vi "ICDAS_Main.vi"() -> ()   [LabVIEW 2018]
doc: "This is the central application/framework that controls module, run scripts, etc"
uses:
  Framework/InstrumentModulesControl.ctl
  SubVI/VisualizationManagement/PopInOutButton.ctl
  SubVI/Power Request Master 2012 NIVerified/Power Availabilty Requests/Type Defs/Power Request Type.ctl
  NistPluggableModules/BusClass/Bus.lvclass/Bus.ctl
  TypeDefs/PythonOrINIScript.ctl
  LV_Config_class/Typedefs/eLogLvl.ctl
  SubVI/VisualizationManagement/VisualizationManagerActions.ctl
  LV_Config_class/Config.lvclass/Config.ctl
  LV_TestAutomation/Comms_lib/CommsData.ctl
  NistPluggableModules/TestClass/Test.lvclass
  NistPluggableModules/TestClass/Test.lvclass/Test.ctl
  NistPluggableModules/BusClass/Accessors/Read Test.vi
  LV_Config_class/Accessors/Read ConfigFilePath.vi
  NistPluggableModules/TestClass/Accessors/Write ModuleIDs.vi
  <extravilib>/ChannelInstances/Tag-bool/Read With Abort.vi
  <extravilib>/ChannelInstances/Tag-bool/Write With Abort.vi
  <extravilib>/ChannelInstances/Tag-bool/Instantiate.vi
  <extravilib>/ChannelInstances/Tag-bool/EndpointRead.vi
  SubVI/Message Queue/Enqueue Message (Single).vi
  <vilib>/Utility/error.llb/Error Cluster From Error Code.vi
  <extravilib>/ChannelInstances/Tag-bool/Endpoint.vi
  <vilib>/ErrorRing/Error Ring.xnode
  Queue/Queue.lvlib
  <userlib>/NIST/NISTErrorLib/NISTErrorLib.lvlib
  LV_Config_class/Config.lvclass
  <vilib>/Utility/config.llb/NI_LVConfig.lvlib
  LV_Ini/Ini_lib.lvlib
  NistPluggableModules/BusClass/Bus.lvclass
  NistPluggableModules/Visualization/Visualization.lvlib
  LV_TestAutomation/Comms_lib/Comms.lvlib
  <extravilib>/ChannelInstances/Tag-bool.lvlib
  LV_TestAutomation/LV-PY_Lib/LV-PY.lvlib
  NistPluggableModules/Visualization/VisualizeBase/VisualizeBase_class/VisualizeBase.lvclass
  SubVI/Message Queue/Message Queue.lvlib
  SubVI/Power Request Master 2012 NIVerified/Power Requests.lvlib
panel:
  in  "btnRunAll":bool
  in  "btnLoadTDMSData":bool
  in  "btnLoadTDMSData":bool
  in  "btnShutdownICDAS":bool
  in  "btnSettings":bool
  in  "btnHide":bool=TRUE
  in  "rngRunningModules":string(combo)
  in  "btnStopOneModule":bool
  in  "btnPopOutModVis":T1
  in  "ICDAS Logo":enum32{"Page 1"}(tab)
  in  "Visualize":bool
  in  "btnClose Visulizations":bool
  in  "btnPlugins":bool
  in  "Instrument Modules":T2=[{"PluginSelection"=4, "ConfigDialog"=FALSE}] {"PluginSelection" items=["C37.118 PMU", "C37.118 Sim", "Base PMU", "RoomAlert0", "RoomAlert1", "RoomAlert0", "RoomAlert1", "none", "SiemensDEM0"]}
  in  "Experiment Specific Controls":T3(tab)
  in  "Priority":u8=2
  in  "Severity":string="Abort"
  out "COMMS Loop":bool
  in  "RelativePathToINIFiles":string[](array[string])=["..\\UserFiles\\Plugins\\Sensor"]
  in  "Tool Bar?":bool
  out "Error Out":errorcluster
  in  "Severity":string
  in  "Priority":u8=2
  in  "Create Error (Test AutoTimeout)":bool
  in  "Error In 2":errorcluster
  in  "btnCreateScriptlet":bool
  in  "btnRunSpecificScript":bool
  out "CurrentLogFile":string
  # "ICDAS"
  # "Integrated Control and Data Acquisition System"
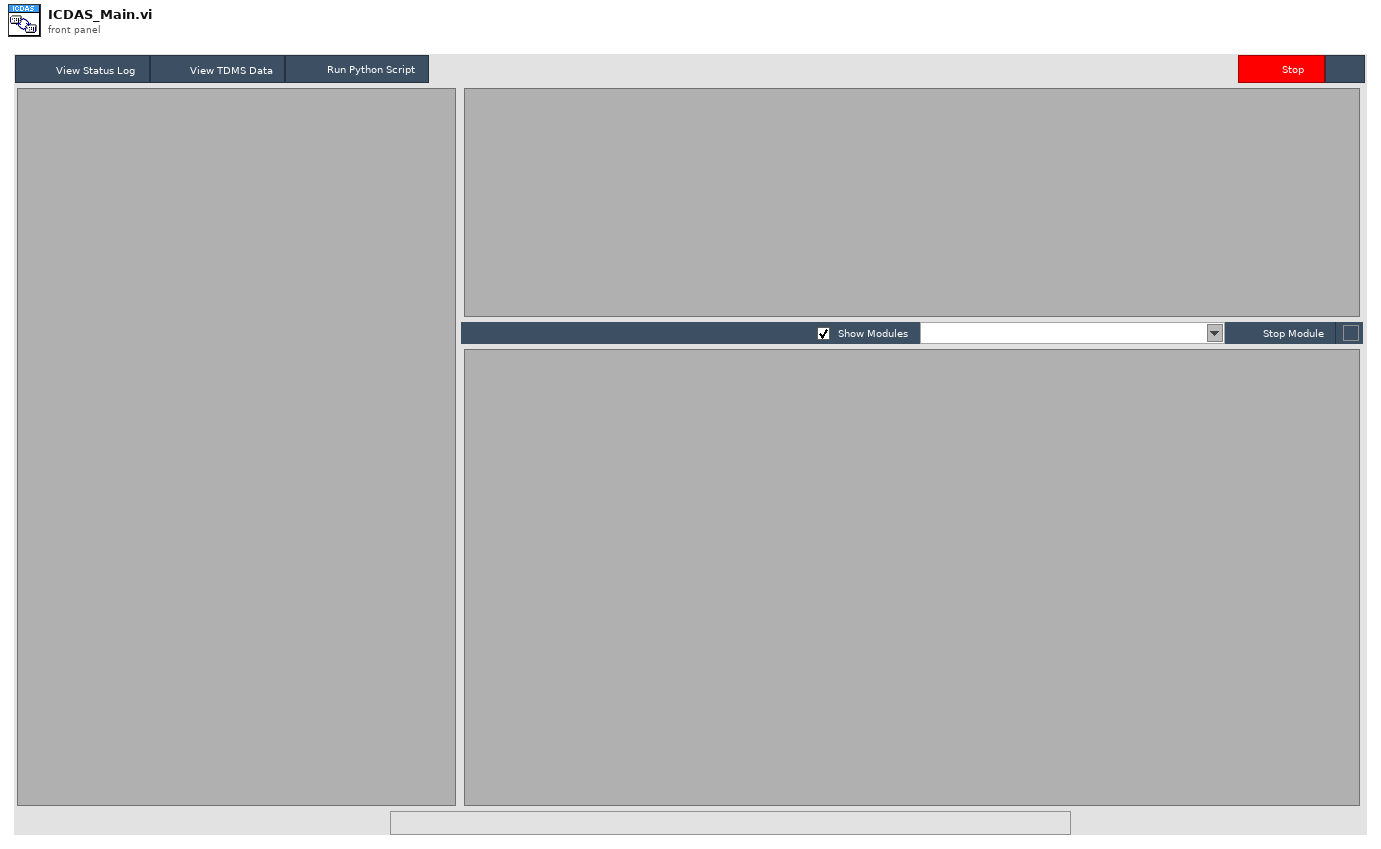
[diagram p1: front panel]
types:
  T1 = typedef "PopInOutButton.ctl" = bool
  T2 = typedef "InstrumentModulesControl.ctl" = cluster{"PluginSelection":u16, "ConfigDialog":bool}[]
  T3 = enum32{"PV Aging Experiment", "Pacific Power ", "Miscellaneous ", "Errors", "Test AutoTimeout", "Test Python MutliRun"}
  T4 = typedef "Power Requests.lvlib/Power Request Type.ctl" = enum32{"Power Request Display Required", "Power Request System Required", "Power Request Away Mode Required", "Power Request Execution Required"}
  T5 = typedef "clUserEvents.ctl" = cluster{"StopEvent":refnum<user-event>, "RefreshUserEvents":refnum<user-event>, "StatusUpdate":refnum<user-event>, "RunAllScripts":refnum<user-event>}
  T6 = typedef "DigitizerShared.lvlib/clBroadcastEvents.ctl" = cluster{"DidInit":refnum<user-event>, "StatusUpdate":refnum<user-event>, "ErrorReport":refnum<user-event>, "DidStop":refnum<user-event>, "PathToINI":refnum<user-event>, "Channels":refnum<user-event>, "Acq":refnum<user-event>, "Trigger":refnum<user-event>, "Waveforms":refnum<user-event>}
  T7 = typedef "FgenShared.lvlib/clBroadcastEvents.ctl" = cluster{"DidInit":refnum<user-event>, "StatusUpdate":refnum<user-event>, "ErrorReport":refnum<user-event>, "DidStop":refnum<user-event>, "PathToINI":refnum<user-event>, "Channels":refnum<user-event>, "Function":refnum<user-event>, "Waveforms":refnum<user-event>, "Triggers":refnum<user-event>, "FunctionParams":refnum<user-event>, "FunctionArbs":refnum<user-event>, "FunctionSampleRate":refnum<user-event>}
  T8 = typedef "SyncModule.lvlib/SyncBroadcastEvents.ctl" = cluster{"DidInit":refnum<user-event>, "StatusUpdate":refnum<user-event>, "ErrorReport":refnum<user-event>, "DidStop":refnum<user-event>, "PathToINI":refnum<user-event>, "TriggerTime":refnum<user-event>, "LockStatus":refnum<user-event>, "Info":refnum<user-event>, "ClockProperties":refnum<user-event>, "SyncData":refnum<user-event>}
  T9 = typedef "AnalysisModule.lvlib/clBroadcastEvents.ctl" = cluster{"DidInit":refnum<user-event>, "StatusUpdate":refnum<user-event>, "ErrorReport":refnum<user-event>, "DidStop":refnum<user-event>, "PathToINI":refnum<user-event>, "Config":refnum<user-event>, "ResultReport":refnum<user-event>, "FunctionClass":refnum<user-event>, "State":refnum<user-event>, "FunctionParams":refnum<user-event>, "Duration":refnum<user-event>}
  T10 = typedef "SensorShared.lvlib/clBroadcastEvents.ctl" = cluster{"DidInit":refnum<user-event>, "StatusUpdate":refnum<user-event>, "ErrorReport":refnum<user-event>, "DidStop":refnum<user-event>, "PathToINI":refnum<user-event>, "SensorReport":refnum<user-event>, "SensorConfig":refnum<user-event>}
  T11 = typedef "ScopeShared.lvlib/clBroadcastEvents.ctl" = cluster{"DidInit":refnum<user-event>, "StatusUpdate":refnum<user-event>, "ErrorReport":refnum<user-event>, "DidStop":refnum<user-event>, "PathToINI":refnum<user-event>, "Handle":refnum<user-event>, "Model":refnum<user-event>, "Channels":refnum<user-event>, "Acquisition":refnum<user-event>, "Trigger":refnum<user-event>, "ExtAcquisition":refnum<user-event>, "Waveform":refnum<user-event>}
  T12 = typedef "AcPwrShared.lvlib/AcPwrBroadcastEvents.ctl" = cluster{"DidInit":refnum<user-event>, "StatusUpdate":refnum<user-event>, "ErrorReport":refnum<user-event>, "DidStop":refnum<user-event>, "PathToINI":refnum<user-event>, "Measurements":refnum<user-event>, "LoadConfigFile":refnum<user-event>, "GetSettings":refnum<user-event>, "SetSettings":refnum<user-event>, "GetType&ID":refnum<user-event>, "GotSettings":refnum<user-event>}
  T13 = cluster{"DigitizerEvents":T6, "FGenEvents":T7, "SyncBroadcastEvents":T8, "AnalysisBroadcastEvents":T9, "SensorBdcstEvents":T10, "ScopeEvents":T11, "clAcPwrEvents":T12}
  T14 = typedef "Visualization.lvlib/VisualizeBase.lvclass/VisBroadcastEvents.ctl" = cluster{"WindowMinimized":refnum<user-event>, "WindowClosed":refnum<user-event>}
  T15 = typedef "cntlRefs.ctl" = cluster{"rngFGen":refnum<vi>, "rngDigitizer":refnum<vi>, "btnHide":refnum<vi>, "rngInst":refnum<vi>, "Instrument Modules":refnum<vi>, "RelativePathToINIFiles ":refnum<vi>, "PluginTree":refnum<vi>, "TestListboxRef":refnum<vi>, "path.tstFile":refnum<vi>, "cmbxRunningModules":refnum<vi>, "TestDataSubPanel":refnum<vi>, "TestDataCaption":refnum<vi>, "btnPopInOut":refnum<vi>, "PluginMgrQ":refnum<queue>, "TestMgrQ":refnum<queue>, "TestMgrSubPanel":refnum<vi>, "PluginMgrSubPanel":refnum<vi>, "PwrReqHandle":u32, "btnStopOneTest":refnum<vi>, "pathUserfiles":refnum<vi>, "PluginTreeCaption":refnum<vi>, "MainVIRef":refnum<vi>}
  T16 = typedef "Comms.lvlib/CommsData.ctl" = cluster{"Command":string, "XMLData":string}
  T17 = typedef "VisualizationManagerActions.ctl" = enum16{"Set", "LoadModVI", "PopInOutModVI", "Add", "Clear", "CloseVisMod", "LoadLatestModule"}
  T18 = typedef "NI_LVConfig.lvlib/Config Data RefNum.ctl" = refnum<k1>
  T19 = typedef "LVBoundsTypeDef.ctl" = cluster{"Width":u32, "Height":u32}
  T20 = typedef "Tag-bool.lvlib/))Channel.ctl" = refnum<queue>
  T21 = typedef "PythonOrINIScript.ctl" = enum16{"INIScript", "Python"}
  T22 = typedef "Config_class.lvlib/Config.lvclass/eLogLvl.ctl" = enum16{"Normal", "Verbose", "None"}
  T23 = enum32{"Invalid", "Standard", "Closed", "Hidden", "Minimized", "Maximized"}
  T24 = typedef "Config_class.lvlib/Config.lvclass/RootDir.ctl" = cluster{"pathRootDir":path, "btnOutPath":bool, "OutDir":string, "btnOpenOutputDir":bool, "ScriptDir":string, "btnOpenScriptDir":bool, "TestDir":string, "btnOpenTestDir":bool}
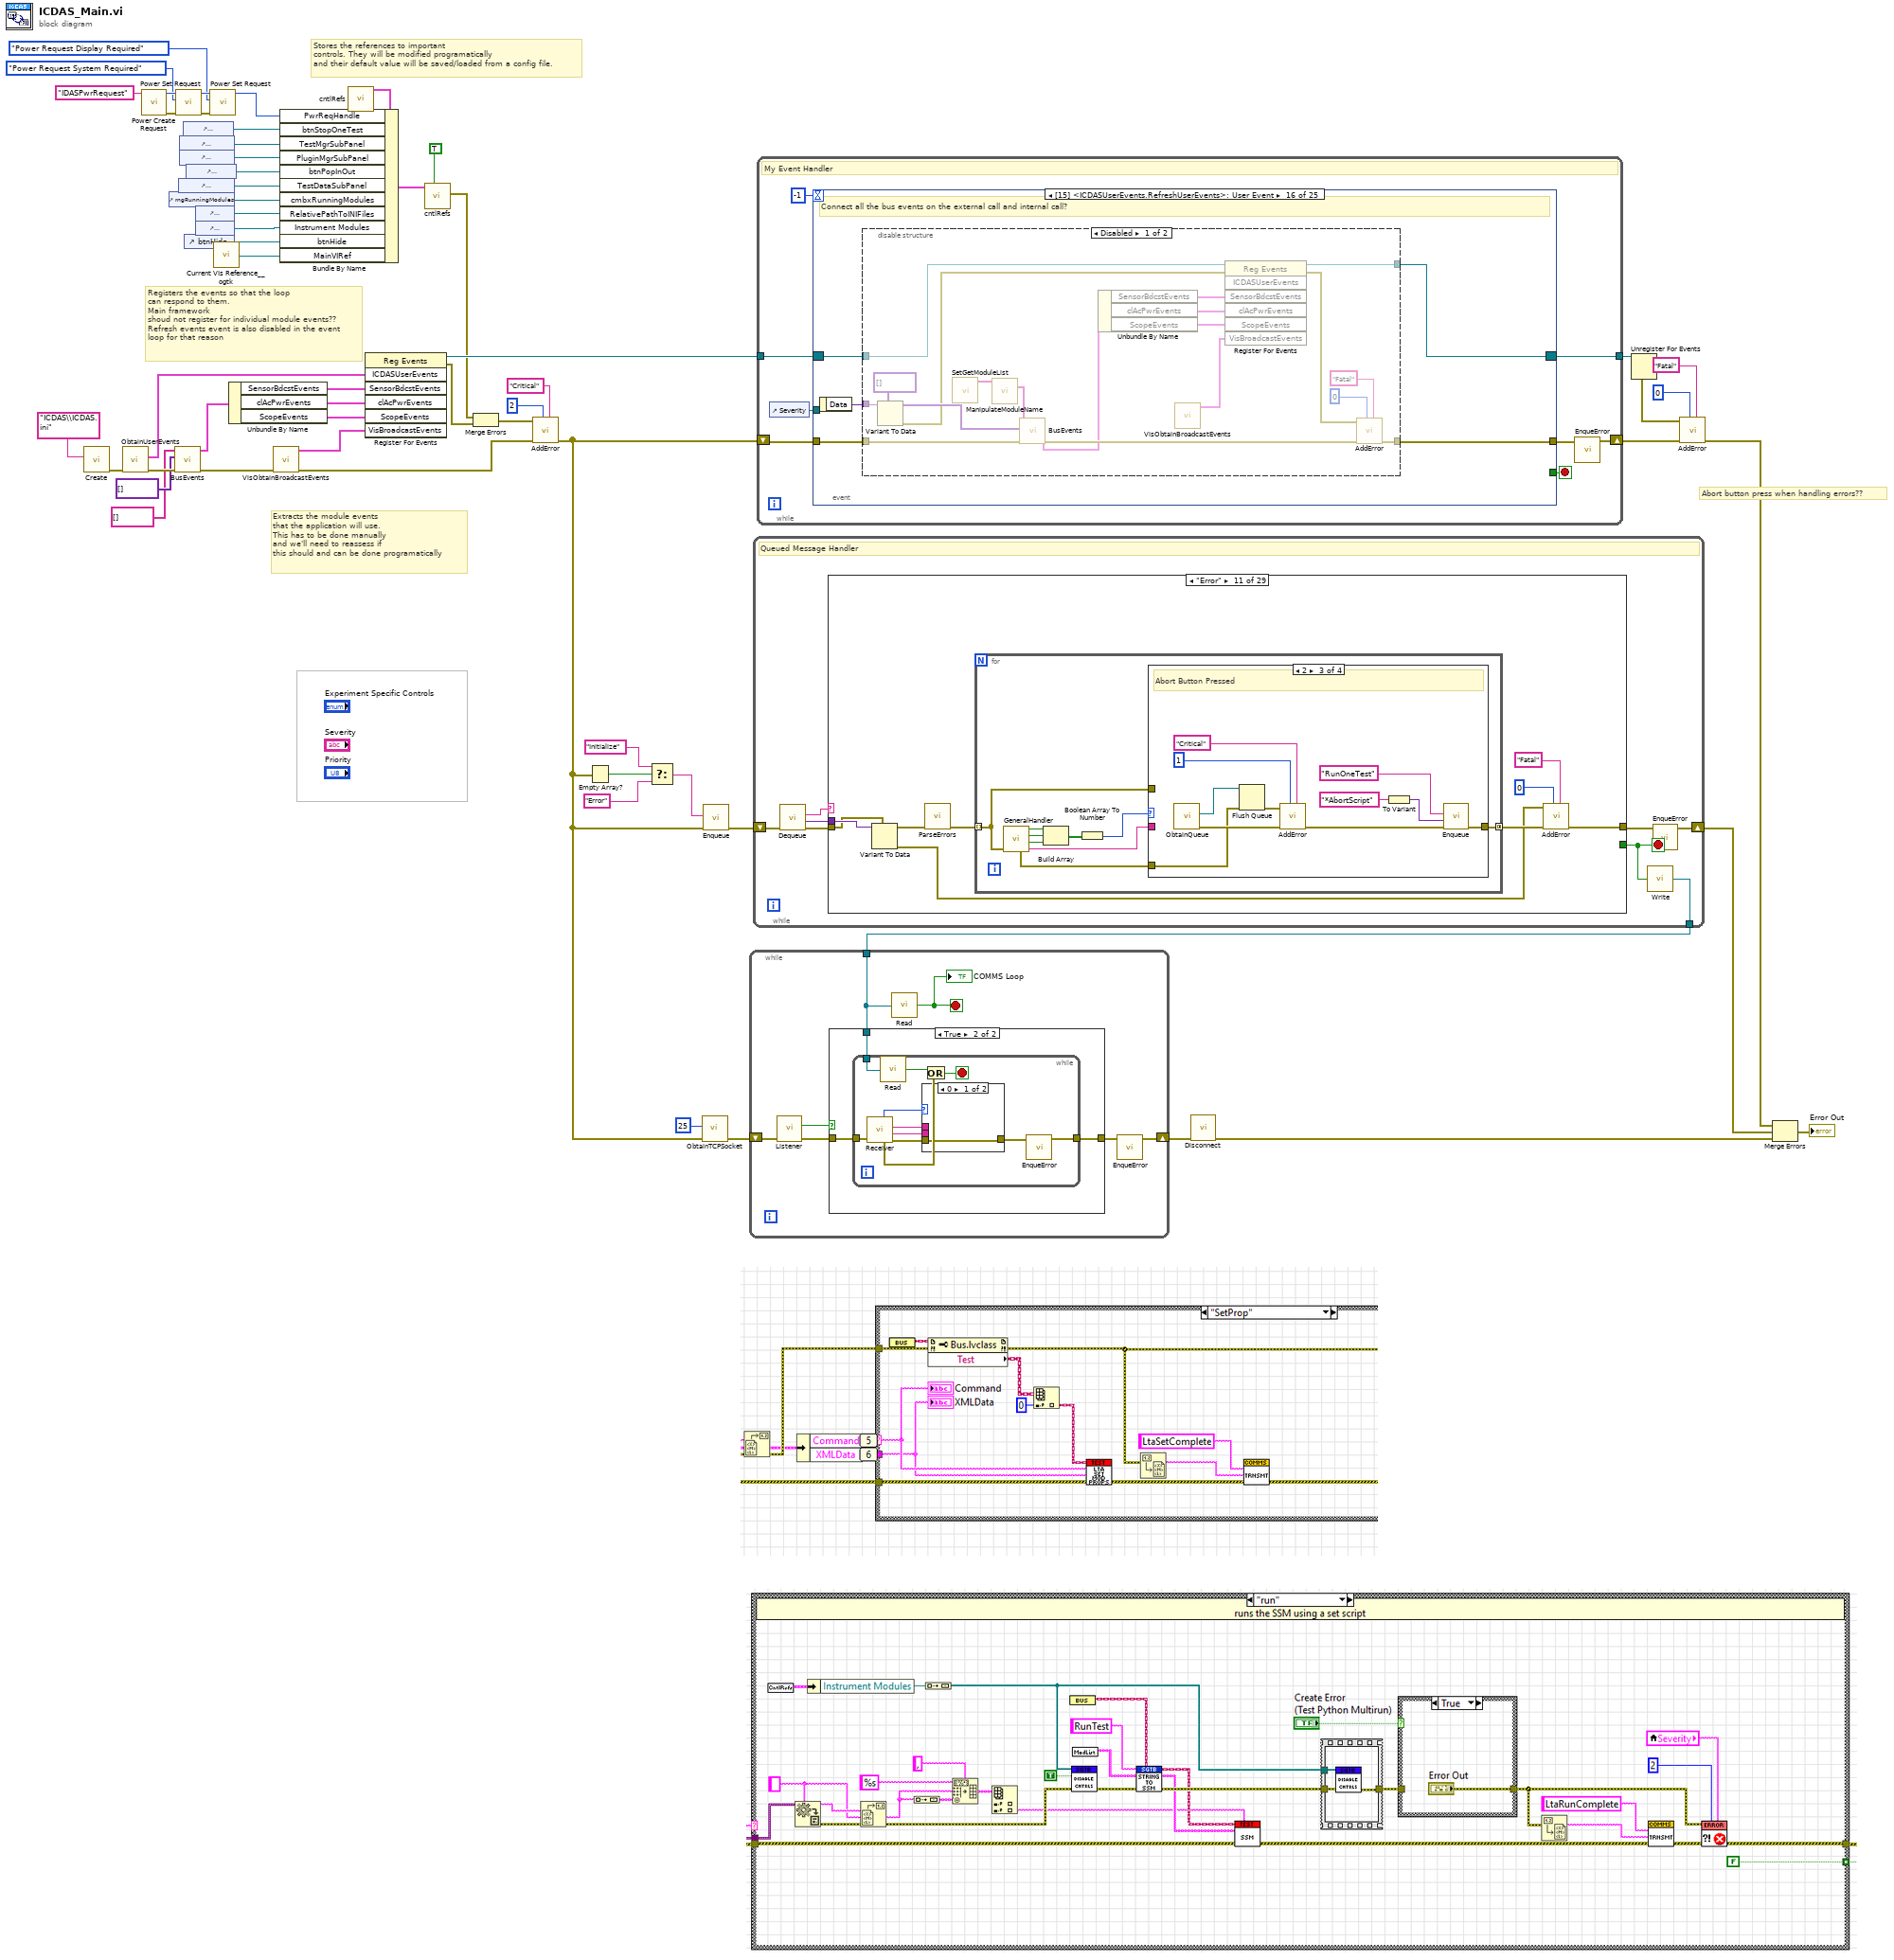
[diagram p0: block diagram]
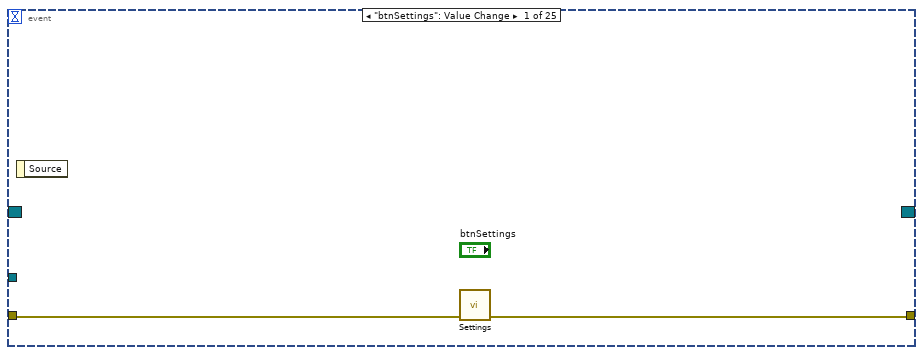
[diagram p2: hidden frame]
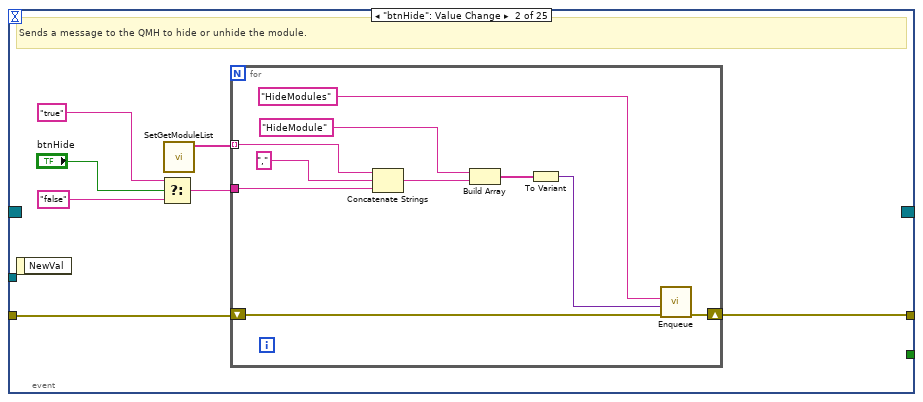
[diagram p3: hidden frame]
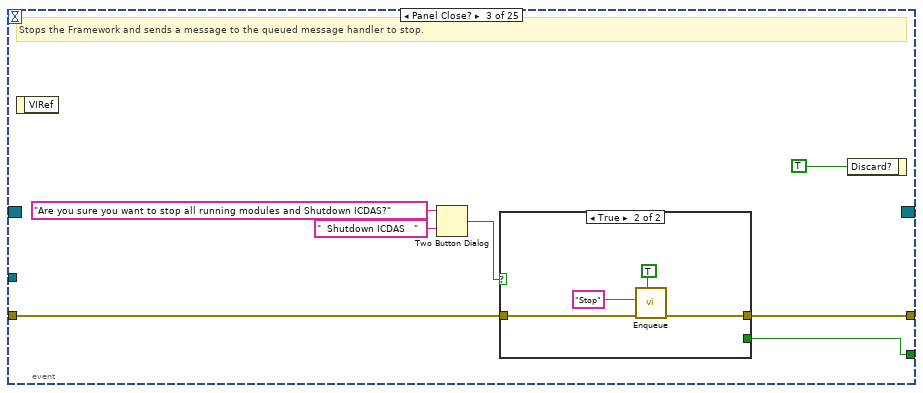
[diagram p4: hidden frame]
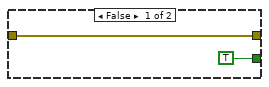
[diagram p5: hidden frame]
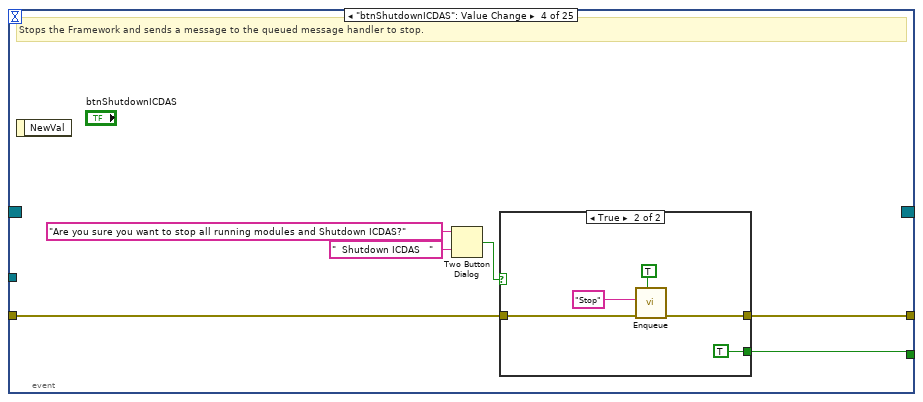
[diagram p6: hidden frame]
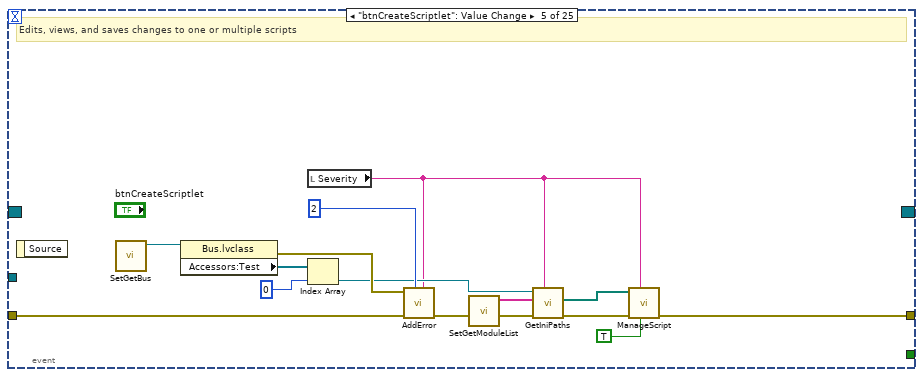
[diagram p8: hidden frame]
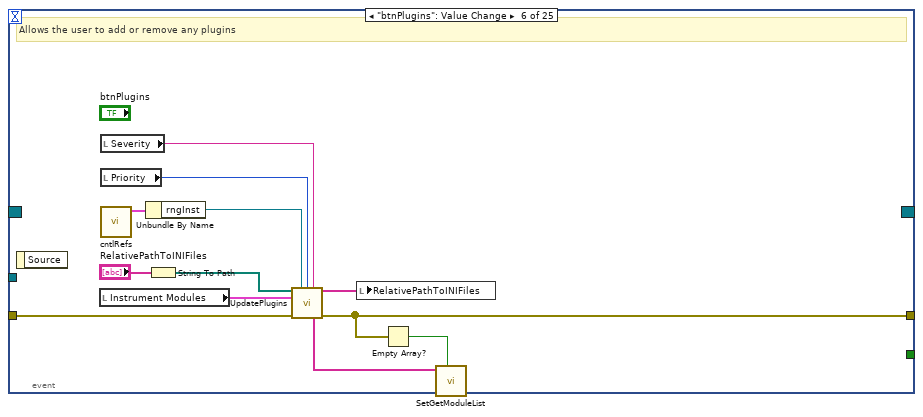
[diagram p9: hidden frame]
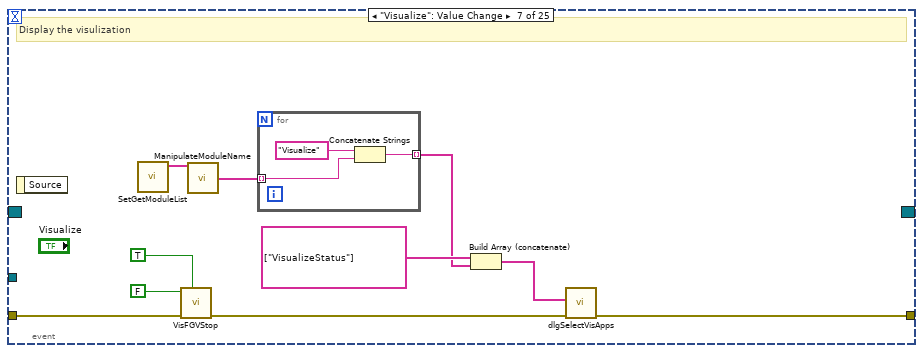
[diagram p10: hidden frame]
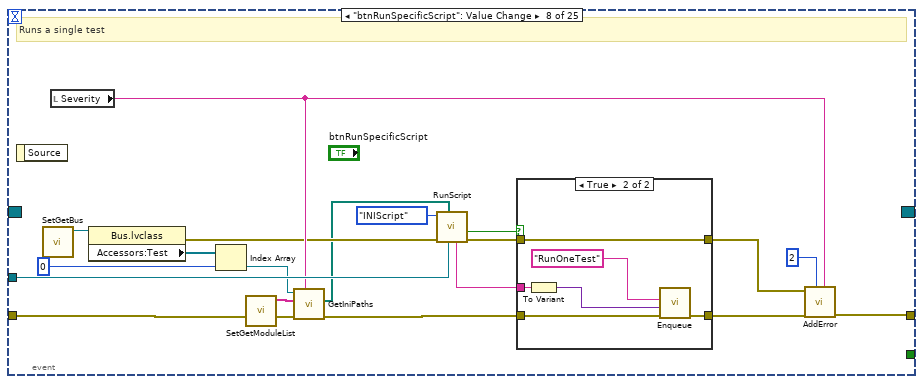
[diagram p11: hidden frame]
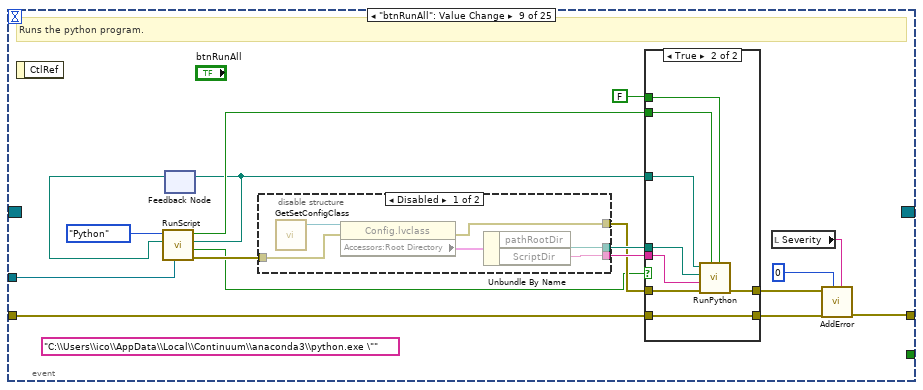
[diagram p13: hidden frame]
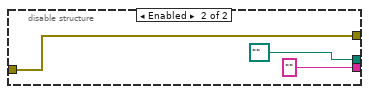
[diagram p15: hidden frame]
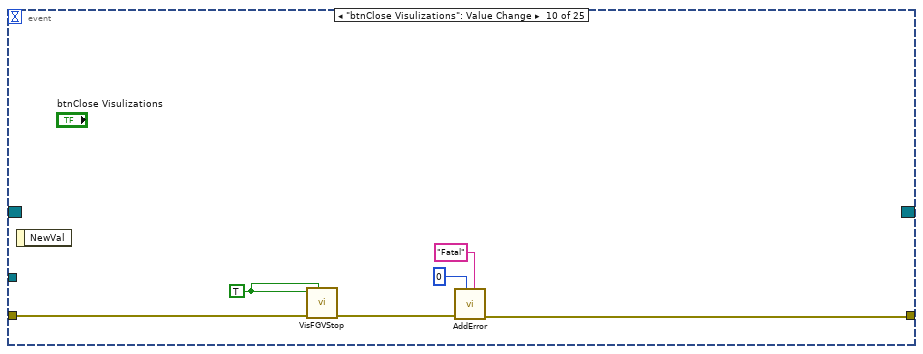
[diagram p16: hidden frame]
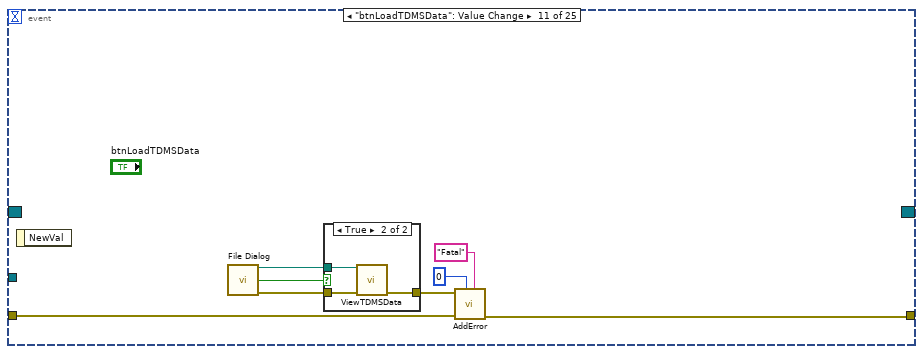
[diagram p17: hidden frame]
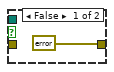
[diagram p18: hidden frame]
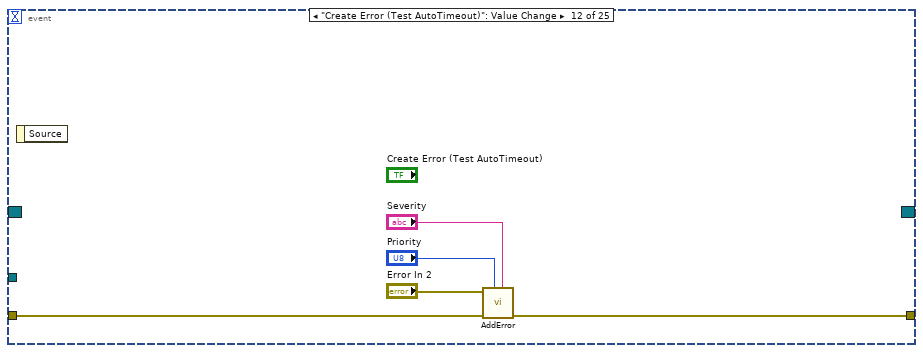
[diagram p19: hidden frame]
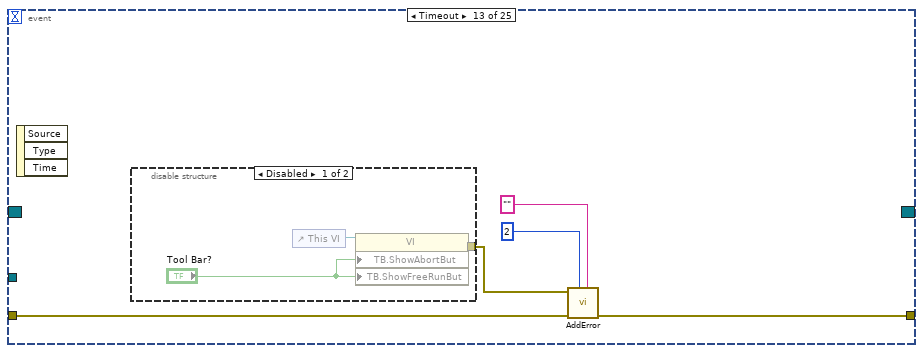
[diagram p20: hidden frame]
diagram:
  # "Abort button press when handling errors??"
  # "Registers the events so that the loop \ncan respond to them.\nMain framework\nshoud not register for individual module events??\nRefresh events event is also disabled in the event \nloop for that reason"
  # "Extracts the module events\nthat the application will use. \nThis has to be done manually \nand we'll need to reassess if \nthis should and can be done programatically"
  # "Stores the references to important\ncontrols. They will be modified programatically\nand their default value will be saved/loaded from a config file."
  n1 = call "Create.vi"("name or relative path"="ICDAS\\ICDAS.ini") -> ("ErrorArray"=w51:errorcluster[])  [unwired: 9 in, 1 out]
  n2 = call "ObtainUserEvents.vi"("ErrorArray"=w51) -> ("ErrorArray"=w52:errorcluster[], "ICDASUserEvents"=w58:T5)  [unwired: 9 in]
  n3 = call "Power Create Request.vi"("Simple Reason String"="IDASPwrRequest") -> ("error out"=w16:errorcluster, "Handle"=w17:i64)  [unwired: 9 in]
  n4 = control-ref of="rngRunningModules"() -> (w25:refnum<vi>)
  n5 = call "BusEvents.vi"("Error in"=w52, "EventArray"=variant[] [], "ModuleList"=string[] []) -> ("Error out"=w9:errorcluster[], "output cluster"=w39:T13)  [unwired: 7 in]
  n6 = call "Power Set Request.vi"("error in (no error)"=w16, "Power Request Type"=Power_Request_Type."Power Request System Required", "Handle in"=w17) -> ("error out"=w14:errorcluster, "Handle out"=w15:u32)  [unwired: 6 in, 1 out]
  n7 = control-ref of="TestDataSubPanel"() -> (w24:refnum<vi>)
  n8 = control-ref of="TestMgrSubPanel"() -> (w19:refnum<vi>)
  n9 = control-ref of="PluginMgrSubPanel"() -> (w20:refnum<vi>)
  n10 = control-ref of="btnStopOneModule"() -> (w10:refnum<vi>)
  n11 = control-ref of="btnHide"() -> (w48:refnum<vi>)
  n12 = control-ref of="btnPopOutModVis"() -> (w23:refnum<vi>)
  n13 = control-ref of="RelativePathToINIFiles"() -> (w34:refnum<vi>)
  n14 = control-ref of="Instrument Modules"() -> (w37:refnum<vi>)
  n15 = call "Power Set Request.vi"("error in (no error)"=w14, "Power Request Type"=Power_Request_Type."Power Request Display Required", "Handle in"=w15) -> ("Handle out"=w11:u32)  [unwired: 6 in, 2 out]
  n16 = call <userlib>:"Current VIs Reference__ogtk.vi"() -> ("Current VI's reference"=w1:refnum<vi>)  [unwired: 5 in]
  n17 = Unbundle By Name(w39) -> ("SensorBdcstEvents"=w38:T10, "clAcPwrEvents"=w4:T12, "ScopeEvents"=w29:T11)
  n18 = call "VisObtainBroadcastEvents.vi"("Error"=w9) -> ("Error"=w8:errorcluster[], "VisBroadcastEvents"=w3:T14)  [unwired: 9 in]
  n19 = call "cntlRefs.vi"() -> ("cntlRefs"=w22:T15)  [unwired: 10 in, 1 out]
  n20 = Bundle By Name(cluster=w22, "PwrReqHandle"=w11, "btnStopOneTest"=w10, "TestMgrSubPanel"=w19, "PluginMgrSubPanel"=w20, "btnPopInOut"=w23, "TestDataSubPanel"=w24, "cmbxRunningModules"=w25, "RelativePathToINIFiles"=w34, "Instrument Modules"=w37, "btnHide"=w48, "MainVIRef"=w1) -> (w41:T15)
  n21 = register-events(w58, w38, w4, w29, w3) -> (reference out=w59:refnum<event-registration>, error out=w28:errorcluster)  [unwired: 2 in]
  n22 = call "cntlRefs.vi"("Set?"=TRUE, "cntlRefs"=w41) -> ("error out"=w26:errorcluster[])  [unwired: 8 in, 1 out]
  n23 = Merge Errors(w26, w28) -> (w27:errorcluster)
  n24 = call <userlib>:"AddError.vi"("Severity"="Critical", "Priority"=u8 2, "ErrorArray In"=w8, "error in (no error)"=w27) -> ("ErrorArray Out"=w40:errorcluster[])  [unwired: 6 in, 1 out]
  n25 = Empty Array?(array=w40) -> (empty?=w56:bool)
  n26 = Select(t="Initialize" ("Message"), s=w56, f="Error") -> (s? t:f=w53:string)
  n27 = call "ObtainTCPSocket.vi"("ErrorArray"=w40, "timeout"=25) -> ("ErrorArray"=w46:errorcluster[])  [unwired: 8 in, 1 out]
  n28 = call "Enqueue.vi"("ErrorArray"=w40, "Message"=w53) -> ("ErrorArray"=w57:errorcluster[])  [unwired: 9 in]
  n29 = while {
    shift-right: [w64] -> w35
    shift-left: w57 -> [w67]
    tunnel: [w60] -> w43
    stop <- w62 stop-if-true
    # "Queued Message Handler"
    n30 = call "Dequeue.vi"("ErrorArray"=w67) -> ("ErrorArray"=w63:errorcluster[], "Message Data"=w61:variant, "Message"=w66:string)  [unwired: 8 in]
    n31 = case shown="\"Error\"" w66 {
      selector: w66 -> [_ _ _ _ _ _ _ _ _ _ _ _ _ _ _ _ w306 _ _ _ _ _ _ _ _ _ _ _ _]
      tunnel: [w68 w82 w91 w107 w129 w130 w137 w153 w214 w216 w218 w249 w256 w262 w283 w297 w305 w314 w329 w331 w338 w341 w347 w352 w354 w361 w371 w375 w397] -> w65
      tunnel: w63 -> [w68 w70 w101 w114 w128 w130 w139 w154 w215 w216 w223 w255 w256 w261 w278 w300 w304 w314 w330 w331 w337 w346 w347 w351 w354 w361 w371 w374 w397]
      tunnel: [_ _ _ _ _ _ _ _ _ _ _ _ _ _ _ TRUE _ _ _ _ _ _ _ _ _ _ _ _ _] -> w62
      tunnel: w61 -> [_ _ _ _ w127 _ w140 w155 _ _ w224 w254 _ _ w282 _ _ _ w327 _ w336 _ _ _ _ _ w365 w381 _]
      frame "----Initialization----" {
      }
      frame "Initialize" {
        # "Pulls the default configuration from the INI file"
        n32 = call "GetSetConfigClass.vi"() -> ("Ref out"=w87:refnum<class "Config.lvclass">)  [unwired: 11 in]
        n33 = property class="Config.lvclass"(reference=w87) -> ("Accessors:ConfigFilePath"=w84:path)  [unwired: 1 in, 2 out]
        n34 = call "Enqueue.vi"("ErrorArray"=w70, "Message"="Load Manager VIs") -> ("ErrorArray"=w69:errorcluster[])  [unwired: 9 in]
        n35 = To Variant(anything=w84) -> (Variant=w83:variant)
        n36 = call "Enqueue.vi"("ErrorArray"=w69, "Message Data"=w83, "Message"="LoadTest") -> ("ErrorArray"=w72:errorcluster[])  [unwired: 8 in]
        n37 = call "ClearBus.vi"("ErrorIn"=w72) -> ("ErrorOut"=w73:errorcluster[])  [unwired: 10 in]
        n38 = call "Enqueue.vi"("ErrorArray"=w73, "Message Data"=FALSE, "Message"="Clear Test Controls") -> ("ErrorArray"=w74:errorcluster[])  [unwired: 8 in]
        n39 = call "Enqueue.vi"("ErrorArray"=w74, "Message Data"=FALSE ("Delete Children?"), "Message"="Show Test Data Controls") -> ("ErrorArray"=w79:errorcluster[])  [unwired: 8 in]
        n40 = call "Enqueue.vi"("ErrorArray"=w79, "Message"="Center Logo") -> ("ErrorArray"=w81:errorcluster[])  [unwired: 9 in]
        n41 = call <userlib>:"AddError.vi"("Severity"="Fatal", "Priority"=u8 0, "ErrorArray In"=w81) -> ("ErrorArray Out"=w82:errorcluster[])  [unwired: 7 in, 1 out]
      }
      frame "Load Manager VIs" {
        # "Load Plugin Manager first..."
        n42 = call "cntlRefs.vi"() -> ("cntlRefs"=w100:T15)  [unwired: 10 in, 1 out]
        n43 = Unbundle By Name(w100) -> ("PluginMgrSubPanel"=w95:refnum<vi>)
        n44 = vi-ref "PluginManager.vi"() -> (w96:refnum<vi>)
        n45 = invoke class="VI" method="FP.Close"(reference=w96) -> (reference out=w97:refnum<vi>)  [unwired: 2 in, 2 out]
        n46 = invoke class="VI" method="Run VI"(reference=w97, "Wait until done"=FALSE ("Wait Until Done"), "Auto Dispose Ref"=FALSE ("Auto Dispose Reference")) -> (reference out=w93:refnum<vi>, error out=w94:errorcluster)  [unwired: 2 in, 3 out]
        n47 = invoke class="SubPnl" method="Insert VI"(reference=w95, error in=w94, "VI Ref"=w93) -> (error out=w92:errorcluster)  [unwired: 1 in, 3 out]
        n48 = call <userlib>:"AddError.vi"("Severity"="Fatal", "Priority"=u8 0, "ErrorArray In"=w101, "error in (no error)"=w92) -> ("ErrorArray Out"=w91:errorcluster[])  [unwired: 6 in, 1 out]
      }
      frame "Plugin Manager Loaded" {
        # "Load Test Manager after plugin manager has been loaded"
        n49 = vi-ref "TestManager.vi"() -> (w113:refnum<vi>)
        n50 = call "cntlRefs.vi"() -> ("cntlRefs"=w104:T15)  [unwired: 10 in, 1 out]
        n51 = invoke class="VI" method="FP.Close"(reference=w113) -> (reference out=w112:refnum<vi>)  [unwired: 2 in, 2 out]
        n52 = Unbundle By Name(w104) -> ("TestMgrSubPanel"=w103:refnum<vi>)
        n53 = invoke class="VI" method="Run VI"(reference=w112, "Wait until done"=FALSE ("Wait Until Done"), "Auto Dispose Ref"=FALSE ("Auto Dispose Reference")) -> (reference out=w111:refnum<vi>, error out=w110:errorcluster)  [unwired: 2 in, 3 out]
        n54 = invoke class="SubPnl" method="Insert VI"(reference=w103, error in=w110, "VI Ref"=w111) -> (error out=w102:errorcluster)  [unwired: 1 in, 3 out]
        n55 = call <userlib>:"AddError.vi"("Severity"="Critical", "Priority"=u8 2, "ErrorArray In"=w114, "error in (no error)"=w102) -> ("ErrorArray Out"=w107:errorcluster[])  [unwired: 6 in, 1 out]
      }
      frame "LoadTest" {
        # "From the default file load the last saved results and updated the controls and indicators"
        n56 = call "cntlRefs.vi"() -> ("cntlRefs"=w121:T15)  [unwired: 10 in, 1 out]
        n57 = Unbundle By Name(w121) -> ("btnHide"=w120:refnum<vi>)
        n58 = Variant To Data(type=path "", Variant=w127) -> (data=w123:path, error out=w125:errorcluster)  [unwired: 1 in]
        n59 = call <vilib>:"Open Config Data.vi"("error in (no error)"=w125, "configuration file path"=w123) -> ("error out"=w117:errorcluster, "refnum"=w122:T18)  [unwired: 7 in, 1 out]
        n60 = Build Array(w120) -> (w119:refnum<vi>[])
        n61 = call "InitBoolValues.vi"("ErrorArray in"=w128, "BoolRefArray"=w119, "IniFileRef in"=w122) -> ("ErrorArray Out"=w126:errorcluster[], "IniFileRef out"=w118:T18)  [unwired: 7 in]
        n62 = call <vilib>:"Close Config Data.vi"("error in (no error)"=w117, "refnum"=w118) -> ("error out"=w116:errorcluster)  [unwired: 8 in, 1 out]
        n63 = call <userlib>:"AddError.vi"("Severity"="Inform", "ErrorArray In"=w126, "error in (no error)"=w116) -> ("ErrorArray Out"=w129:errorcluster[])  [unwired: 7 in, 1 out]
      }
      frame "----Python Communications----" {
      }
      frame "get" {
        n64 = Variant To Data(type="", Variant=w140) -> (data=w133:string, error out=w132:errorcluster)  [unwired: 1 in]
        n65 = call "GetSetTestClass.vi"() -> ("Test.lvclass"=w131:refnum<class "Test.lvclass">)  [unwired: 11 in]
        n66 = local read "Severity"() -> (w134:string)
        n67 = call "LtaGetModuleProperties.vi"("Error In"=w139, "arg"=w133, "Test.lvclass"=w131) -> ("Error Out"=w135:errorcluster[])  [unwired: 6 in, 2 out]
        n68 = call <userlib>:"AddError.vi"("Severity"=w134, "Priority"=u8 2, "ErrorArray In"=w135, "error in (no error)"=w132) -> ("ErrorArray Out"=w137:errorcluster[])  [unwired: 6 in, 1 out]
      }
      frame "set" {
        # "Different kinds of set commands"
        n69 = Variant To Data(type="", Variant=w155) -> (data=w150:string, error out=w149:errorcluster)  [unwired: 1 in]
        n70 = Unflatten From XML(xml string=w150, type=T16 {"Command"="", "XMLData"=""} ("CommsData"), error in (no error)=w149) -> (value=w151:T16, error out=w142:errorcluster)
        n71 = Unbundle By Name(w151) -> ("Command"=w144:string, "XMLData"=w145:string)
        n72 = case shown="\"everythingelse\", Default" w144 {
          selector: w144 -> [w161 w195 _]
          tunnel: w154 -> [w165 w200 w213]
          tunnel: [w163 w201 w212] -> w146
          tunnel: w145 -> [w162 w198 _]
          tunnel: [w160 w206 w211] -> w143
          tunnel: w142 -> [w157 w199 w211]
          frame "everythingelse", Default {
            # "All other cases"
            n73 = call "GetSetTestClass.vi"() -> ("Test.lvclass"=w156:refnum<class "Test.lvclass">)  [unwired: 11 in]
            n74 = disable-structure shown="Disabled" {
              disable-tunnel: w165 -> [w174 w191]
              disable-tunnel: [w173 w192] -> w164
              disable-tunnel: w162 -> [w172 w188]
              disable-tunnel: w161 -> [w171 w189]
              disable-tunnel: [w168 w193] -> w160
              disable-tunnel: w157 -> [w167 w193]
              disable-tunnel: w156 -> [w166 w190]
              frame Disabled {
                n75 = call "ArgumentManipulation.vi"("String"=w171) -> ("Argument"=w169:string, "Property or SSM"=w170:string)  [unwired: 9 in]
                n76 = case shown="\"SSM\", Default" w170 {
                  tunnel: w174 -> [w181 w187]
                  tunnel: [w180 w186] -> w173
                  tunnel: w172 -> [_ w185]
                  tunnel: w169 -> [w177 w184]
                  tunnel: w167 -> [w176 w183]
                  tunnel: [w176 w183] -> w168
                  tunnel: w166 -> [w175 w182]
                  frame "SSM", Default {
                    n77 = Build Array(w177, "Stop") -> (w178:string[])
                    n78 = call "ScriptedStateMachine.vi"("ErrorArray"=w181, "script"=w178, "Test.lvclass"=w175) -> ("ErrorArray"=w180:errorcluster[])  [unwired: 6 in, 2 out]
                  }
                  frame "Prop" {
                    n79 = call "LtaSetModuleProperties.vi"("Error In"=w187, "XmlData"=w185, "Arg"=w184, "Test.lvclass"=w182) -> ("Error Out"=w186:errorcluster[])  [unwired: 6 in, 1 out]
                  }
                }
              }
              frame Enabled {
                n80 = call "LtaSetModuleProperties.vi"("Error In"=w191, "XmlData"=w188, "Arg"=w189, "Test.lvclass"=w190) -> ("Error Out"=w192:errorcluster[])  [unwired: 6 in, 1 out]
              }
            }
            n81 = Flatten To XML(anything=w160) -> (xml string=w158:string)
            n82 = call "Transmitter.vi"("ErrorArray"=w164, "XMLData"=w158, "Command"="LtaSetComplete") -> ("ErrorArray"=w163:errorcluster[])  [unwired: 7 in, 1 out]
          }
          frame "RunTest" {
            # "If the python script want to cause a plugin to run a script in its file."
            n83 = Unflatten From XML(xml string=w198, type=w198, error in (no error)=w199) -> (value=w196:string, error out=w197:errorcluster)
            n84 = Flatten To XML(anything=w197) -> (xml string=w204:string)
            n85 = call "Transmitter.vi"("ErrorArray"=w200, "XMLData"=w204, "Command"="LtaSetComplete") -> ("ErrorArray"=w202:errorcluster[])  [unwired: 7 in, 1 out]
            n86 = call "SetGetModuleList.vi"() -> ("ModuleList"=w205:string[])  [unwired: 11 in]
            n87 = call "SetGetBus.vi"() -> ("Bus.lvclass"=w208:refnum<class "Bus.lvclass">)  [unwired: 11 in]
            n88 = call "GetSetTestClass.vi"() -> ("Test.lvclass"=w194:refnum<class "Test.lvclass">)  [unwired: 11 in]
            n89 = call "StringToSSM.vi"("Bus Reference"=w208, "Error Out"=w197, "ModuleList"=w205, "SSM Case"=w195) -> ("Error Out 2"=w206:errorcluster, "SSM Array"=w207:string[])  [unwired: 6 in]
            n90 = call "ScriptedStateMachine.vi"("ScriptSectionName"=w196, "ErrorArray"=w202, "script"=w207, "Test.lvclass"=w194) -> ("ErrorArray"=w201:errorcluster[])  [unwired: 5 in, 2 out]
          }
          frame "handshake" {
            # "If Python wants to establish if the framework is ready for further commands"
            n91 = Flatten To XML(anything=w211) -> (xml string=w209:string)
            n92 = call "Transmitter.vi"("ErrorArray"=w213, "XMLData"=w209, "Command"="LtaSetComplete") -> ("ErrorArray"=w212:errorcluster[])  [unwired: 7 in, 1 out]
          }
        }
        n93 = local read "Severity"() -> (w141:string)
        n94 = call <userlib>:"AddError.vi"("Severity"=w141, "Priority"=u8 2, "ErrorArray In"=w146, "error in (no error)"=w143) -> ("ErrorArray Out"=w153:errorcluster[])  [unwired: 6 in, 1 out]
      }
      frame "run" {
        # "Run all test scripts per \"run\" request from Python"
        # "runs the SSM using a set script"
        n95 = call "RunAllScripts.vi"("ErrorArray"=w215) -> ("ErrorArray"=w214:errorcluster[])  [unwired: 10 in]
      }
      frame "----Handle Errors----" {
      }
      frame "Error" {
        n96 = Variant To Data(type=w223, Variant=w224) -> (data=w222:errorcluster[], error out=w217:errorcluster)  [unwired: 1 in]
        n97 = call <userlib>:"ParseErrors.vi"("ErrorArray"=w222) -> ("ErrorArray"=w225:errorcluster[])  [unwired: 8 in, 2 out]
        n98 = for {
          tunnel: w225 -> [w231] mode=indexing
          tunnel: [w234] -> w219 mode=concatenating
          n99 = call <userlib>:"GeneralHandler.vi"("error in (no error)"=w231) -> ("Severity"=w232:string, "Stop"=w228:bool, "Abort"=w229:bool, "Continue"=w230:bool, "Error Out"=w226:errorcluster)  [unwired: 6 in]
          n100 = Build Array(w230, w229, w228) -> (w227:bool[])
          n101 = Boolean Array To Number(Boolean array=w227) -> (number=w233:u32)
          n102 = case shown="2" w233 {
            tunnel: w232 -> [_ _ _ _]
            tunnel: [_ _ w236 w246] -> w234
            tunnel: w231 -> [_ _ _ _]
            tunnel: w226 -> [_ _ w240 _]
            frame 0, Default {
              # "No Dialog"
            }
            frame 1 {
              # "Continue"
            }
            frame 2 {
              # "Abort Button Pressed"
              n103 = call "ObtainQueue.vi"() -> ("ErrorArray"=w243:errorcluster[], "QueueRef"=w245:refnum<queue>)  [unwired: 10 in]
              n104 = Flush Queue(queue=w245, error in (no error)=w240) -> (error out=w244:errorcluster)  [unwired: 2 out]
              n105 = call <userlib>:"AddError.vi"("Severity"="Critical", "Priority"=u8 1, "ErrorArray In"=w243, "error in (no error)"=w244) -> ("ErrorArray Out"=w237:errorcluster[])  [unwired: 6 in, 1 out]
              n106 = To Variant(anything="*AbortScript" ("Message")) -> (Variant=w238:variant)
              n107 = call "Enqueue.vi"("ErrorArray"=w237, "Message Data"=w238, "Message"="RunOneTest") -> ("ErrorArray"=w236:errorcluster[])  [unwired: 8 in]
            }
            frame 4 {
              # "Stop this application"
              n108 = call "StopEvent.vi"() -> ("ErrorArray"=w246:errorcluster[])  [unwired: 11 in]
            }
          }
        }
        n109 = call <userlib>:"AddError.vi"("Severity"="Fatal", "Priority"=u8 0, "ErrorArray In"=w219, "error in (no error)"=w217) -> ("ErrorArray Out"=w218:errorcluster[])  [unwired: 6 in, 1 out]
      }
      frame "ClientError" {
        n110 = Variant To Data(type="", Variant=w254) -> (data=w252:string, error out=w247:errorcluster)  [unwired: 1 in]
        n111 = Unflatten From XML(xml string=w252, type=w247, error in (no error)=w247) -> (value=w248:errorcluster, error out=w250:errorcluster)
        n112 = call <userlib>:"AddError.vi"("ErrorArray In"=w255, "error in (no error)"=w250) -> ("ErrorArray Out"=w251:errorcluster[])  [unwired: 8 in, 1 out]
        n113 = Build Array (concatenate)(w251, w248) -> (w249:errorcluster[])
      }
      frame "----Exiting Application----" {
      }
      frame "Stop" {
        n114 = call "GetSetConfigClass.vi"() -> ("Ref out"=w265:refnum<class "Config.lvclass">)  [unwired: 11 in]
        n115 = property class="Config.lvclass"(reference=w265) -> (error out=w259:errorcluster, "Accessors:ConfigFilePath"=w258:path)  [unwired: 1 in, 1 out]
        n116 = local read "Severity"() -> (w257:string)
        n117 = call "Enqueue.vi"("ErrorArray"=w261, "Message Data"=w258, "Message"="SaveTest") -> ("ErrorArray"=w260:errorcluster[])  [unwired: 8 in]
        n118 = call <userlib>:"AddError.vi"("Severity"=w257, "Priority"=u8 0, "ErrorArray In"=w260, "error in (no error)"=w259) -> ("ErrorArray Out"=w262:errorcluster[])  [unwired: 6 in, 1 out]
      }
      frame "SaveTest" {
        # "Save Show Modules boolean value for next run"
        # "saves the state of the controls and indicators into an INI file"
        n119 = call "cntlRefs.vi"() -> ("cntlRefs"=w274:T15)  [unwired: 10 in, 1 out]
        n120 = Variant To Data(type=path "", Variant=w282) -> (data=w277:path, error out=w281:errorcluster)  [unwired: 1 in]
        n121 = Unbundle By Name(w274) -> ("btnHide"=w272:refnum<vi>)
        n122 = call <vilib>:"Open Config Data.vi"("error in (no error)"=w281, "configuration file path"=w277) -> ("error out"=w280:errorcluster, "refnum"=w276:T18)  [unwired: 7 in, 1 out]
        n123 = call <userlib>:"AddError.vi"("ErrorArray In"=w278, "error in (no error)"=w280) -> ("ErrorArray Out"=w279:errorcluster[])  [unwired: 8 in, 1 out]
        n124 = Build Array(w272) -> (w271:refnum<vi>[])
        n125 = call "BoolsToIni.vi"("ErrorArray in"=w279, "BoolRefArray"=w271, "IniFileRef in"=w276) -> ("ErrorArray out"=w267:errorcluster[], "InifileRef out"=w268:T18)  [unwired: 7 in]
        n126 = call <vilib>:"Close Config Data.vi"("write file if changed (T)"=TRUE, "refnum"=w268) -> ("error out"=w270:errorcluster)  [unwired: 8 in, 1 out]
        n127 = call <userlib>:"AddError.vi"("ErrorArray In"=w267, "error in (no error)"=w270) -> ("ErrorArray Out"=w266:errorcluster[])  [unwired: 8 in, 1 out]
        n128 = call "Enqueue.vi"("ErrorArray"=w266, "Message"="End") -> ("ErrorArray"=w283:errorcluster[])  [unwired: 9 in]
      }
      frame "End" {
        w291 = TRUE ("Priority Message? (F)")
        w292 = "Stop" ("Severity")
        n129 = call "StopEvent.vi"("ErrorArray"=w300) -> ("ErrorArray"=w298:errorcluster[])  [unwired: 10 in]
        n130 = local write "CurrentLogFile"("") -> ()
        n131 = call "cntlRefs.vi"() -> ("cntlRefs"=w296:T15)  [unwired: 10 in, 1 out]
        n132 = Unbundle By Name(w296) -> ("PwrReqHandle"=w286:u32, "PluginMgrQ"=w294:refnum<queue>, "TestMgrQ"=w293:refnum<queue>)
        n133 = call "CloseQueue.vi"("ErrorArray"=w298) -> ("ErrorArray 2"=w297:errorcluster[])  [unwired: 10 in]
        n134 = call-poly "Enqueue Message.vi"("Priority Message? (F)"=w291, "Message"=w292, "Message Queue"=w293) -> ()  [unwired: 7 in, 2 out]
        n135 = call-poly "Enqueue Message.vi"("Priority Message? (F)"=w291, "Message"=w292, "Message Queue"=w294) -> ()  [unwired: 7 in, 2 out]
        n136 = call "Power Clear Request.vi"("Power Request Type"=Power_Request_Type."Power Request System Required", "Handle in"=w286) -> ("error out"=w289:errorcluster, "Handle out"=w290:u32)  [unwired: 7 in, 1 out]
        n137 = call "Power Clear Request.vi"("error in (no error)"=w289, "Power Request Type"=Power_Request_Type."Power Request Display Required", "Handle in"=w290) -> ("error out"=w287:errorcluster, "Handle out"=w288:u32)  [unwired: 6 in, 1 out]
        n138 = call "Close Handle.vi"("error in (no error)"=w287, "Handle"=w288) -> ()  [unwired: 8 in, 2 out]
      }
      frame Default {
        n139 = xnode "Error Ring"("parameter 0"=w306) -> ("error out"=w301:errorcluster)
        n140 = call <userlib>:"AddError.vi"("Severity"="Inform", "Priority"=u8 5, "ErrorArray In"=w304, "error in (no error)"=w301) -> ("ErrorArray Out"=w305:errorcluster[])  [unwired: 6 in, 1 out]
      }
      frame "----UI Events----" {
      }
      frame "HideModules" {
        # "runs the SSM using a set script"
        n141 = Variant To Data(type=string[] [], Variant=w327) -> (data=w320:string[], error out=w328:errorcluster)  [unwired: 1 in]
        n142 = Index Array(array=w320) -> (element #1=w318:string, element #2=w319:string)  [unwired: 2 in]
        n143 = Build Array(w319) -> (w317:string[])
        n144 = call "SetGetBus.vi"() -> ("Bus.lvclass"=w323:refnum<class "Bus.lvclass">)  [unwired: 11 in]
        n145 = call "StringToSSM.vi"("Bus Reference"=w323, "Error Out"=w328, "ModuleList"=w317, "SSM Case"=w318) -> ("Error Out 2"=w321:errorcluster, "SSM Array"=w322:string[])  [unwired: 6 in]
        n146 = call "GetSetTestClass.vi"() -> ("Test.lvclass"=w315:refnum<class "Test.lvclass">)  [unwired: 11 in]
        n147 = call "ScriptedStateMachine.vi"("ErrorArray"=w330, "script"=w322, "Test.lvclass"=w315) -> ("ErrorArray"=w324:errorcluster[])  [unwired: 6 in, 2 out]
        n148 = local read "Severity"() -> (w316:string)
        n149 = call <userlib>:"AddError.vi"("Severity"=w316, "Priority"=u8 2, "ErrorArray In"=w324, "error in (no error)"=w321) -> ("ErrorArray Out"=w329:errorcluster[])  [unwired: 6 in, 1 out]
      }
      frame "----Messages From Test Manager----" {
      }
      frame "Test Started" {
        n150 = Variant To Data(type=path "", Variant=w336) -> (data=w332:path)  [unwired: 1 in, 1 out]
        n151 = Format Into String(format string="%s (Click to Open)", w332) -> (resulting string=→"CurrentLogFile":string)  [unwired: 2 in, 1 out]
        n152 = call "Enqueue.vi"("ErrorArray"=w337, "Message Data"=TRUE ("Delete Children?"), "Message"="Show Test Data Controls") -> ("ErrorArray"=w338:errorcluster[])  [unwired: 8 in]
      }
      frame "All Tests Stopped" {
        n153 = call "Enqueue.vi"("ErrorArray"=w346, "Message"="Clear Test Controls") -> ("ErrorArray"=w342:errorcluster[])  [unwired: 9 in]
        n154 = call "Enqueue.vi"("ErrorArray"=w342, "Message Data"=FALSE ("Delete Children?"), "Message"="Show Test Data Controls") -> ("ErrorArray"=w341:errorcluster[])  [unwired: 8 in]
      }
      frame "----Messages to Test Manager----" {
      }
      frame "Stop One Module" {
        n155 = local read "rngRunningModules"() -> (w348:string)
        n156 = call "cntlRefs.vi"() -> ("cntlRefs"=w353:T15)  [unwired: 10 in, 1 out]
        n157 = Unbundle By Name(w353) -> ("TestMgrQ"=w350:refnum<queue>)
        n158 = call-poly "Enqueue Message.vi"("error in (no error)"=w351, "Message Data"=w348, "Message"="Stop One Module", "Message Queue"=w350) -> ("error out"=w352:errorcluster[])  [unwired: 6 in, 1 out]
      }
      frame "----Test Data Visualization----" {
      }
      frame "Center Logo" {
        w355 = 2.0
        n159 = property on="Visualization Pane" class="Pane"() -> ("Bounds"=w356:T19)  [unwired: 2 in, 2 out]
        n160 = property on="ICDAS Logo" class="TabCtl (strict)"() -> ("Bounds"=w360:T19)  [unwired: 2 in, 2 out]
        n161 = Divide(x=w356, y=w355) -> (x/y=w357:cluster{"Width":dbl, "Height":dbl})
        n162 = Divide(x=w360, y=w355) -> (x/y=w359:cluster{"Width":dbl, "Height":dbl})
        n163 = Subtract(x=w357, y=w359) -> (x-y=w358:cluster{"Width":dbl, "Height":dbl})
        n164 = property on="ICDAS Logo" class="TabCtl (strict)"("Position"=w358) -> ()  [unwired: 2 in, 2 out]
      }
      frame "Show Test Data Controls" {
        n165 = Variant To Data(type=FALSE ("Visible"), Variant=w365) -> (data=w362:bool)  [unwired: 1 in, 1 out]
        n166 = call "cntlRefs.vi"() -> ("cntlRefs"=w370:T15)  [unwired: 10 in, 1 out]
        n167 = Unbundle By Name(w370) -> ("TestDataCaption"=w369:refnum<vi>, "btnHide"=w368:refnum<vi>, "cmbxRunningModules"=w367:refnum<vi>, "btnPopInOut"=w366:refnum<vi>, "btnStopOneTest"=w363:refnum<vi>)
        n168 = property class="Str"(reference=w369, "Visible"=w362) -> ()  [unwired: 1 in, 2 out]
        n169 = property class="Bool (strict)"(reference=w368, "Visible"=w362) -> ()  [unwired: 1 in, 2 out]
        n170 = property class="CmbBox"(reference=w367, "Visible"=w362) -> ()  [unwired: 1 in, 2 out]
        n171 = property class="Bool"(reference=w366, "Visible"=w362) -> ()  [unwired: 1 in, 2 out]
        n172 = property class="Bool"(reference=w363, "Visible"=w362) -> ()  [unwired: 1 in, 2 out]
      }
      frame "Pop In or Out of SubPanel" {
        n173 = Variant To Data(type=cluster{"Module Name":string, "In SubPanel?":T1} {"Module Name"="", "In SubPanel?"=FALSE} ("output cluster"), Variant=w381) -> (data=w379:cluster{"Module Name":string, "In SubPanel?":T1}, error out=w376:errorcluster)  [unwired: 1 in]
        n174 = Unbundle(w379) -> ("Module Name"=w378:string, "In SubPanel?"=w377:T1)
        n175 = call "VisualizationManager.vi"("Action"=VisualizationManagerActions."PopInOutModVI", "error in (no error)"=w376, "Load In SubPanel?"=w377, "Module Name"=w378) -> ("error out"=w382:errorcluster, "In SubPanel?"=w372:bool, "Module Name out"=w373:string)  [unwired: 4 in, 1 out]
        n176 = local write "rngRunningModules"(w373) -> ()
        n177 = local write "btnPopOutModVis"(w372) -> ()
        n178 = call <userlib>:"AddError.vi"("Severity"="Critical", "Priority"=u8 2, "ErrorArray In"=w374, "error in (no error)"=w382) -> ("ErrorArray Out"=w375:errorcluster[])  [unwired: 6 in, 1 out]
      }
      frame "Clear Test Controls" {
        w394 = refnum<class "Test.lvclass"> refnum  # Test.lvclass
        n179 = call "cntlRefs.vi"() -> ("cntlRefs"=w391:T15)  [unwired: 10 in, 1 out]
        n180 = Unbundle By Name(w391) -> ("cmbxRunningModules"=w388:refnum<vi>, "TestDataSubPanel"=w390:refnum<vi>)
        n181 = call "SetGetModuleList.vi"("Set? (F)"=TRUE) -> ()  [unwired: 10 in, 1 out]
        n182 = call "VisualizationManager.vi"("Action"=VisualizationManagerActions."Clear") -> ()  [unwired: 7 in, 4 out]
        n183 = invoke class="SubPnl" method="Remove VI"(reference=w390) -> ()  [unwired: 2 in, 3 out]
        n184 = property class="CmbBox"(reference=w388, "Strings[]"=string[] [] ("Strings []")) -> ()  [unwired: 1 in, 2 out]
        n185 = property class="Test.lvclass"(reference=w394, "Accessors:ModuleIDs"=i32[] [] ("ModuleIDs")) -> (reference out=w396:refnum<class "Test.lvclass">)  [unwired: 1 in, 1 out]
        n186 = local write "CurrentLogFile"("") -> ()
        n187 = call "GetSetTestClass.vi"("Set"=TRUE, "Test.lvclass"=w396) -> ()  [unwired: 9 in, 1 out]
      }
    }
    n188 = call <extravilib>:"Write.vi"("element"=w62) -> ("channel"=w60:T20)  [unwired: 1 out]
    n189 = call "EnqueError.vi"("ErrorArrayIn"=w65) -> ("ErrorArrayOut"=w64:errorcluster[])  [unwired: 10 in]
  }
  n190 = while {
    shift-right: [w400] -> w45
    shift-left: w46 -> [w404]
    tunnel: w43 -> [w398]
    stop <- w399 stop-if-true
    n191 = call "Listener.vi"("ErrorArray"=w404) -> ("ErrorArray"=w403:errorcluster[], "Accepted?"=w402:bool)  [unwired: 9 in]
    n192 = case shown="True" w402 {
      tunnel: w403 -> [w406 w409]
      tunnel: [w406 w408] -> w401
      tunnel: w398 -> [_ w407]
      frame False {
        n193 = Wait (ms)(milliseconds to wait=u32 10) -> ()  [unwired: 1 out]
      }
      frame True {
        n194 = while {
          tunnel: w409 -> [w420]
          tunnel: [w415] -> w408
          tunnel: w407 -> [w410]
          stop <- w413 stop-if-true
          n195 = call "Receiver.vi"("ErrorArray"=w420) -> ("ErrorArray"=w416:errorcluster[], "XMLData"=w417:string, "Command"=w418:string, "error out"=w412:errorcluster, "bytes_read"=w419:i32)  [unwired: 6 in]
          n196 = call <extravilib>:"Read.vi"("channel"=w410) -> ("element"=w411:bool)  [unwired: 1 in, 1 out]
          n197 = case shown="0" w419 {
            tunnel: w418 -> [_ w422]
            tunnel: w417 -> [_ w426]
            tunnel: w416 -> [w421 w424]
            tunnel: [w421 w425] -> w414
            frame 0 {
            }
            frame 1, Default {
              n198 = To Variant(anything=w426) -> (Variant=w423:variant)
              n199 = call "Enqueue.vi"("ErrorArray"=w424, "Message Data"=w423, "Message"=w422) -> ("ErrorArray"=w425:errorcluster[])  [unwired: 8 in]
            }
          }
          n200 = Or(x=w411, y=w412) -> (x .or. y?=w413:bool)
          n201 = call "EnqueError.vi"("ErrorArrayIn"=w414) -> ("ErrorArrayOut"=w415:errorcluster[])  [unwired: 10 in]
        }
      }
    }
    n202 = call <extravilib>:"Read.vi"("channel"=w398) -> ("element"=w399:bool)  [unwired: 1 in, 1 out]
    "COMMS Loop" <- w399
    n203 = call "EnqueError.vi"("ErrorArrayIn"=w401) -> ("ErrorArrayOut"=w400:errorcluster[])  [unwired: 10 in]
  }
  n204 = while {
    tunnel: w59 -> [w434]
    shift-right: [w431] -> w31
    shift-left: w40 -> [w433]
    tunnel: [w427] -> w7
    stop <- w430 stop-if-true
    # "My Event Handler"
    n205 = control-ref of="Severity"() -> (w429:refnum<vi>)
    n206 = event shown="[15] <ICDASUserEvents.RefreshUserEvents>: User Event" {
      selector: w434 -> [_ _ _ _ _ _ _ _ _ _ _ _ _ _ _ w653 _ _ _ _ _ _ _ _ _]
      dyn-events: [_ _ _ _ _ _ _ _ _ _ _ _ _ _ _ w654 _ _ _ _ _ _ _ _ _] -> w427
      timeout: -1 -> [_ _ _ _ _ _ _ _ _ _ _ _ _ _ _ _ _ _ _ _ _ _ _ _ _]
      tunnel: w433 -> [w436 w443 w460 w472 w486 w503 w511 w527 w554 w583 w591 w602 w606 w619 w642 w652 w679 w683 _ w700 w711 _ _ w734 _]
      tunnel: [w435 w442 w459 w471 w492 w498 w514 w535 w557 w584 w592 w601 w605 w620 w633 w651 w678 w682 w695 w699 w710 _ _ w736 w739] -> w432
      tunnel: [_ _ w454 w467 _ _ _ _ _ _ _ _ _ _ _ _ w677 _ _ _ _ _ _ _ _] -> w430
      tunnel: w429 -> [_ _ _ _ _ _ _ w536 w549 _ _ _ _ _ _ _ _ _ _ _ _ _ _ _ _]
      event "btnSettings": Value Change {
        n207 = event-data() -> ()  [unwired: 1 in, 1 out]
        n208 = call "Settings.vi"("ErrorArray"=w436) -> ("ErrorArray"=w435:errorcluster[])  [unwired: 10 in]
      }
      event "btnHide": Value Change {
        # "Sends a message to the QMH to hide or unhide the module."
        n209 = event-data() -> ()  [unwired: 1 in, 1 out]
        n210 = Select(t="true" ("data string"), s="btnHide", f="false" ("data string")) -> (s? t:f=w437:string)
        n211 = call "SetGetModuleList.vi"() -> ("ModuleList"=w441:string[])  [unwired: 11 in]
        n212 = for {
          tunnel: w441 -> [w452] mode=indexing
          tunnel: w437 -> [w451]
          shift-right: [w450] -> w442
          shift-left: w443 -> [w449]
          n213 = Concatenate Strings(w452, ",", w451) -> (w453:string)
          n214 = Build Array("HideModule", w453) -> (w446:string[])
          n215 = To Variant(anything=w446) -> (Variant=w448:variant)
          n216 = call "Enqueue.vi"("ErrorArray"=w449, "Message Data"=w448, "Message"="HideModules") -> ("ErrorArray"=w450:errorcluster[])  [unwired: 8 in]
        }
      }
      event Panel Close? {
        # "Stops the Framework and sends a message to the queued message handler to stop."
        n217 = event-data() -> ()  [unwired: 1 in, 1 out]
        n218 = Two Button Dialog(message="Are you sure you want to stop all running modules and Shutdown ICDAS?", 2:"  Shutdown ICDAS   " ("T button name (\"OK\")")) -> (T button?=w455:bool)  [unwired: 1 in]
        n219 = case shown="True" w455 {
          tunnel: w460 -> [w462 w466]
          tunnel: [w462 w465] -> w459
          tunnel: [TRUE ("Priority (F)") _] -> w454
          frame False {
          }
          frame True {
            n220 = call "Enqueue.vi"("Priority (F)"=TRUE, "ErrorArray"=w466, "Message"="Stop") -> ("ErrorArray"=w465:errorcluster[])  [unwired: 8 in]
          }
        }
        n221 = event-data("Discard?"=TRUE) -> ()  [unwired: 1 in, 1 out]
      }
      event "btnShutdownICDAS": Value Change {
        # "Stops the Framework and sends a message to the queued message handler to stop."
        n222 = event-data() -> ()  [unwired: 1 in, 1 out]
        n223 = Two Button Dialog(message="Are you sure you want to stop all running modules and Shutdown ICDAS?", 2:"  Shutdown ICDAS   " ("T button name (\"OK\")")) -> (T button?=w468:bool)  [unwired: 1 in]
        n224 = case shown="True" w468 {
          tunnel: w472 -> [w473 w478]
          tunnel: [w473 w477] -> w471
          tunnel: [_ TRUE ("Priority (F)")] -> w467
          frame False {
          }
          frame True {
            n225 = call "Enqueue.vi"("Priority (F)"=TRUE, "ErrorArray"=w478, "Message"="Stop") -> ("ErrorArray"=w477:errorcluster[])  [unwired: 8 in]
          }
        }
      }
      event "btnCreateScriptlet": Value Change {
        # "Edits, views, and saves changes to one or multiple scripts"
        n226 = event-data() -> ()  [unwired: 1 in, 1 out]
        n227 = call "SetGetBus.vi"() -> ("Bus.lvclass"=w489:refnum<class "Bus.lvclass">)  [unwired: 11 in]
        n228 = property class="Bus.lvclass"(reference=w489) -> (error out=w484:errorcluster, "Accessors:Test"=w490:refnum<class "Test.lvclass">[])  [unwired: 1 in, 1 out]
        n229 = local read "Severity"() -> (w480:string)
        n230 = Index Array(array=w490, index=0 ("Test Index (0)")) -> (element=w483:refnum<class "Test.lvclass">)
        n231 = call <userlib>:"AddError.vi"("Severity"=w480, "Priority"=u8 2, "ErrorArray In"=w486, "error in (no error)"=w484) -> ("ErrorArray Out"=w485:errorcluster[])  [unwired: 6 in, 1 out]
        n232 = call "SetGetModuleList.vi"() -> ("ModuleList"=w482:string[])  [unwired: 11 in]
        n233 = call "GetIniPaths.vi"("Severity"=w480, "Error Array In"=w485, "ModuleList"=w482, "Test.lvclass"=w483) -> ("Error Array Out"=w491:errorcluster[], "Script Locations"=w481:path[])  [unwired: 5 in, 1 out]
        n234 = call "ManageScript.vi"("ScriptNameEnum?(F)"=TRUE ("ScriptNameEnum?"), "Severity"=w480, "ErrorIn Array"=w491, "Script Locations"=w481) -> ("ErrorOut Array"=w492:errorcluster[])  [unwired: 6 in]
      }
      event "btnPlugins": Value Change {
        # "Allows the user to add or remove any plugins"
        n235 = event-data() -> ()  [unwired: 1 in, 1 out]
        n236 = local read "Instrument Modules"() -> (w500:T2)
        n237 = local read "Severity"() -> (w493:string)
        n238 = local read "Priority"() -> (w494:u8)
        n239 = call "cntlRefs.vi"() -> ("cntlRefs"=w504:T15)  [unwired: 10 in, 1 out]
        n240 = Unbundle By Name(w504) -> ("rngInst"=w501:refnum<vi>)
        n241 = String To Path(string="RelativePathToINIFiles") -> (path=w497:path[])
        n242 = call "UpdatePlugins.vi"("Current Paths"=w497, "rngInst"=w501, "Priority"=w494, "Severity (Critical)"=w493, "Instrument Modules"=w500, "Error In Array"=w503) -> ("Current Paths"=w502:string[], "PluginTypes"=w495:string[], "Error Out Array"=w498:errorcluster[])  [unwired: 7 in]
        n243 = local write "RelativePathToINIFiles"(w502) -> ()
        n244 = Empty Array?(array=w498) -> (empty?=w496:bool)
        n245 = call "SetGetModuleList.vi"("Set? (F)"=w496, "ModuleList"=w495) -> ()  [unwired: 9 in, 1 out]
      }
      event "Visualize": Value Change {
        # "Display the visulization"
        n246 = event-data() -> ()  [unwired: 1 in, 1 out]
        n247 = call "SetGetModuleList.vi"() -> ("ModuleList"=w509:string[])  [unwired: 11 in]
        n248 = call "VisFGVStop.vi"("Set? (False)"=TRUE ("Value to Set (False)"), "Error In"=w511, "Value to Set (False)"=FALSE) -> ("Error Out"=w510:errorcluster[])  [unwired: 7 in, 1 out]
        n249 = call "ManipulateModuleName.vi"("ModuleListArrayIn"=w509) -> ("BeforeMatchWithoutRedundantEntries:ModuleListArray"=w508:string[])  [unwired: 9 in, 5 out]
        n250 = for {
          tunnel: w508 -> [w516] mode=indexing
          tunnel: [w515] -> w506 mode=indexing
          n251 = Concatenate Strings("Visualize" ("String"), w516) -> (w515:string)
        }
        n252 = Build Array (concatenate)(string[] ["VisualizeStatus"] ("PathsToVisApps"), w506) -> (w505:string[])
        n253 = call "dlgSelectVisApps.vi"("Error In"=w510, "PathsToVisApps"=w505) -> ("Error Out"=w514:errorcluster[])  [unwired: 9 in]
      }
      event "btnRunSpecificScript": Value Change {
        # "Runs a single test"
        n254 = event-data() -> ()  [unwired: 1 in, 1 out]
        n255 = call "SetGetBus.vi"() -> ("Bus.lvclass"=w524:refnum<class "Bus.lvclass">)  [unwired: 11 in]
        n256 = local read "Severity"() -> (w528:string)
        n257 = property class="Bus.lvclass"(reference=w524) -> (error out=w522:errorcluster, "Accessors:Test"=w525:refnum<class "Test.lvclass">[])  [unwired: 1 in, 1 out]
        n258 = Index Array(array=w525, index=0 ("Test Index (0)")) -> (element=w521:refnum<class "Test.lvclass">)
        n259 = call "SetGetModuleList.vi"() -> ("ModuleList"=w529:string[])  [unwired: 11 in]
        n260 = call "GetIniPaths.vi"("Severity"=w528, "Error Array In"=w527, "ModuleList"=w529, "Test.lvclass"=w521) -> ("Error Array Out"=w526:errorcluster[], "Script Locations"=w520:path[])  [unwired: 5 in, 1 out]
        n261 = call "RunScript.vi"("String Reference (Severity)"=w536, "ScriptFileNames"=w520, "Error In"=w522, "Python or INIScript?"=PythonOrINIScript."INIScript") -> ("Error Out"=w519:errorcluster, "Valid File Path"=w530:bool, "INI Script Name Out"=w533:string)  [unwired: 3 in, 2 out]
        n262 = case shown="True" w530 {
          tunnel: w526 -> [w538 w544]
          tunnel: w533 -> [_ w543]
          tunnel: [w538 w542] -> w531
          tunnel: w519 -> [w537 w539]
          tunnel: [w537 w539] -> w518
          frame False {
          }
          frame True {
            n263 = To Variant(anything=w543) -> (Variant=w540:variant)
            n264 = call "Enqueue.vi"("ErrorArray"=w544, "Message Data"=w540, "Message"="RunOneTest") -> ("ErrorArray"=w542:errorcluster[])  [unwired: 8 in]
          }
        }
        n265 = call <userlib>:"AddError.vi"("Severity"=w528, "Priority"=u8 2, "ErrorArray In"=w531, "error in (no error)"=w518) -> ("ErrorArray Out"=w535:errorcluster[])  [unwired: 6 in, 1 out]
      }
      event "btnRunAll": Value Change {
        (unwired) "C:\\Users\\ico\\AppData\\Local\\Continuum\\anaconda3\\python.exe \"" ("command line")
        # "Runs the python program."
        n266 = event-data() -> ()  [unwired: 1 in, 1 out]
        n267 = feedback #1() -> (w545:path)  [unwired: 1 in]
        n268 = call "RunScript.vi"("String Reference (Severity)"=w549, "File Path to Python Script"=w545, "Python or INIScript?"=PythonOrINIScript."Python") -> ("Error Out"=w551:errorcluster, "Valid File Path"=w548:bool, "File Path Control Out"=w546:path, "Python Script Window"=w552:bool)  [unwired: 4 in, 1 out]
        n269 = feedback-in #1(w546) -> ()
        n270 = disable-structure shown="Disabled" {
          disable-tunnel: [w575 "" ("ScriptDir")] -> w561
          disable-tunnel: [w574 path "" ("PathToUserDir")] -> w560
          disable-tunnel: [w573 w578] -> w553
          disable-tunnel: w551 -> [w572 w578]
          frame Disabled {
            n271 = call "GetSetConfigClass.vi"() -> ("Ref out"=w577:refnum<class "Config.lvclass">)  [unwired: 11 in]
            n272 = property class="Config.lvclass"(reference=w577, error in=w572) -> (error out=w573:errorcluster, "Accessors:Root Directory"=w576:T24)  [unwired: 1 out]
            n273 = Unbundle By Name(w576) -> ("pathRootDir"=w574:path, "ScriptDir"=w575:string)
          }
          frame Enabled {
          }
        }
        n274 = case shown="True" w548 {
          tunnel: w561 -> [_ w571]
          tunnel: w560 -> [_ w570]
          tunnel: w552 -> [_ w569]
          tunnel: [w562 w568] -> w559
          tunnel: FALSE ("Specific Python exe Path") -> [_ w567]
          tunnel: w554 -> [w563 w566]
          tunnel: [w563 w566] -> w555
          tunnel: w553 -> [w562 w565]
          tunnel: w546 -> [_ w564]
          frame False {
          }
          frame True {
            n275 = call "RunPython.vi"("PathToScript"=w564, "PathToUserDir"=w570, "ScriptDir"=w571, "error in (no error)"=w565, "keep cmd window open (f)"=w569, "Specific Python exe Path"=w567) -> ("error out"=w568:errorcluster)  [unwired: 3 in, 1 out]
          }
        }
        n276 = local read "Severity"() -> (w550:string)
        n277 = call <userlib>:"AddError.vi"("Severity"=w550, "Priority"=u8 0, "ErrorArray In"=w555, "error in (no error)"=w559) -> ("ErrorArray Out"=w557:errorcluster[])  [unwired: 6 in, 1 out]
      }
      event "btnClose Visulizations": Value Change {
        w581 = TRUE ("Value to Set (False)")
        n278 = event-data() -> ()  [unwired: 1 in, 1 out]
        n279 = call "VisFGVStop.vi"("Set? (False)"=w581, "Error In"=w583, "Value to Set (False)"=w581) -> ("Error Out"=w582:errorcluster[])  [unwired: 7 in, 1 out]
        n280 = call <userlib>:"AddError.vi"("Severity"="Fatal" ("String"), "Priority"=u8 0, "ErrorArray In"=w582) -> ("ErrorArray Out"=w584:errorcluster[])  [unwired: 7 in, 1 out]
      }
      event "btnLoadTDMSData": Value Change {
        n281 = event-data() -> ()  [unwired: 1 in, 1 out]
        n282 = call "File Dialog"() -> ("selected path"=w588:path, "exists"=w587:bool, "error out"=w589:errorcluster)  [unwired: 12 in, 1 out]
        n283 = case shown="True" w587 {
          tunnel: [errorcluster {"status"=FALSE, "code"=0, "source"=""} ("Error Out") w598] -> w590
          tunnel: w589 -> [_ w597]
          tunnel: w588 -> [_ w596]
          frame False {
          }
          frame True {
            n284 = call "ViewTDMSData.vi"("Error In"=w597, "file path"=w596) -> ("Error Out"=w598:errorcluster)  [unwired: 9 in]
          }
        }
        n285 = call <userlib>:"AddError.vi"("Severity"="Fatal" ("String"), "Priority"=u8 0, "ErrorArray In"=w591, "error in (no error)"=w590) -> ("ErrorArray Out"=w592:errorcluster[])  [unwired: 6 in, 1 out]
      }
      event "Create Error (Test AutoTimeout)": Value Change {
        n286 = event-data() -> ()  [unwired: 1 in, 1 out]
        n287 = call <userlib>:"AddError.vi"("Severity"="Severity", "Priority"="Priority", "ErrorArray In"=w602, "error in (no error)"="Error In 2") -> ("ErrorArray Out"=w601:errorcluster[])  [unwired: 6 in, 1 out]
      }
      event Timeout {
        n288 = event-data() -> ()  [unwired: 1 in, 3 out]
        n289 = disable-structure shown="Disabled" {
          disable-tunnel: [w609 _] -> w604
          frame Disabled {
            n290 = control-ref of="This VI"() -> (w611:refnum<vi>)
            n291 = property class="VI"(reference=w611, "TB.ShowAbortBut"="Tool Bar?", "TB.ShowFreeRunBut"="Tool Bar?") -> (error out=w609:errorcluster)  [unwired: 1 in, 1 out]
          }
          frame Enabled {
          }
        }
        n292 = call <userlib>:"AddError.vi"("Severity"="" ("Severity  2"), "Priority"=u8 2 ("Priority  2"), "ErrorArray In"=w606, "error in (no error)"=w604) -> ("ErrorArray Out"=w605:errorcluster[])  [unwired: 6 in, 1 out]
      }
      event Value Change {
        # "Sends a command to open up the preferences dialog or reloads the modules."
        n293 = event-data() -> ("NewVal"=w617:T2, "OldVal"=w623:T2)  [unwired: 1 in]
        n294 = call "cntlRefs.vi"() -> ("cntlRefs"=w626:T15)  [unwired: 10 in, 1 out]
        n295 = local read "Priority"() -> (w613:u8)
        n296 = local read "Severity"() -> (w612:string)
        n297 = Unbundle By Name(w626) -> ("rngInst"=w616:refnum<vi>)
        n298 = call "ConfigDialog.vi"("Severity (Critical)"=w612, "Priority (2)"=w613, "reference"=w616, "ErrorIn Array"=w619, "Instrument Modules New In"=w617) -> ("ErrorOut Array"=w618:errorcluster[], "Instrument Modules Out"=w627:T2)  [unwired: 5 in]
        n299 = local write "Instrument Modules"(w627) -> ()
        n300 = call "PathToINIFiles.vi"() -> ("IniFilePaths Out"=w624:path[])  [unwired: 11 in]
        n301 = call "GetPluginType.vi"("Instrument Modules In New"=w617, "reference"=w616, "Instrument Modules In Old"=w623, "INIFilePaths"=w624, "Compare? (F)"=TRUE, "ErrorArray In"=w618, "Priority (2)"=w613, "Severity (Critical)"=w612) -> ("PluginTypes"=w622:string[], "PluginSelection Changed?"=w614:bool, "ErrorArray Out"=w625:errorcluster[])  [unwired: 3 in, 2 out]
        n302 = call "SetGetModuleList.vi"("Set? (F)"=w614, "ModuleList"=w622) -> ("ModuleList"=w615:string[])  [unwired: 9 in]
        n303 = flat-sequence {
          tunnel: w625 -> [w630]
          tunnel: [w629] -> w620
          tunnel: w615 -> [_]
          tunnel: w614 -> [w628]
          frame #0 {
            n304 = call "LoadPlugin.vi"("ErrorIn Array"=w630, "PluginSelection Changed?"=w628) -> ("ErrorOut Array"=w629:errorcluster[])  [unwired: 9 in]
          }
        }
      }
      event User Event {
        # "Logs and Status Update from the modules"
        n305 = event-data() -> ("Data"=w647:variant)  [unwired: 1 in]
        n306 = Get Date/Time In Seconds() -> (seconds since 1Jan1904=w648:timestamp)
        n307 = Variant To Data(type="", Variant=w647) -> (data=w645:string, error out=w646:errorcluster)  [unwired: 1 in]
        n308 = Get Date/Time String(date format (0)=enum16{"short", "long", "abbreviated"}."short", seconds (now)=w648, want seconds? (F)=TRUE) -> (date string=w635:string, time string=w636:string)
        n309 = Concatenate Strings(w635, "_" ("string"), w636) -> (w634:string)
        n310 = Format Into String(format string="%s: %s \\r", error in=w646, w634, w645) -> (resulting string=w638:string, error out=w632:errorcluster)  [unwired: 1 in]
        n311 = call "LogMessage.vi"("eLogLvl"=eLogLvl."Normal", "Error In"=w632, "LogMessage"=w638) -> ("Error Out"=w631:errorcluster)  [unwired: 8 in]
        n312 = call <userlib>:"AddError.vi"("Severity"="Inform", "Priority"=u8 4, "ErrorArray In"=w642, "error in (no error)"=w631) -> ("ErrorArray Out"=w633:errorcluster[])  [unwired: 6 in, 1 out]
      }
      event User Event {
        # "Connect all the bus events on the external call and internal call?"
        n313 = event-data() -> ("Data"=w655:variant)  [unwired: 1 in]
        n314 = disable-structure shown="Disabled" {
          disable-tunnel: w655 -> [w674 _]
          disable-tunnel: [w673 w676] -> w654
          disable-tunnel: w653 -> [w672 w676]
          disable-tunnel: w652 -> [w667 w675]
          disable-tunnel: [w665 w675] -> w651
          frame Disabled {
            n315 = Variant To Data(type=variant[] [] ("UsrEvents"), Variant=w674) -> (data=w671:variant[], error out=w669:errorcluster)  [unwired: 1 in]
            n316 = call "SetGetModuleList.vi"() -> ("ModuleList"=w660:string[])  [unwired: 11 in]
            n317 = call "ManipulateModuleName.vi"("ModuleListArrayIn"=w660) -> ("BeforeMatch:ModuleListArray"=w662:string[])  [unwired: 9 in, 5 out]
            n318 = call "BusEvents.vi"("Error in"=w667, "EventArray"=w671, "ModuleList"=w662) -> ("Error out"=w666:errorcluster[], "output cluster"=w661:T13)  [unwired: 7 in]
            n319 = Unbundle By Name(w661) -> ("SensorBdcstEvents"=w659:T10, "clAcPwrEvents"=w658:T12, "ScopeEvents"=w657:T11)
            n320 = call "VisObtainBroadcastEvents.vi"() -> ("VisBroadcastEvents"=w656:T14)  [unwired: 10 in, 1 out]
            n321 = register-events(reference=w672, error in=w669, w659, w658, w657, w656) -> (reference out=w673:refnum<event-registration>, error out=w668:errorcluster)  [unwired: 1 in]
            n322 = call <userlib>:"AddError.vi"("Severity"="Fatal", "Priority"=u8 0, "ErrorArray In"=w666, "error in (no error)"=w668) -> ("ErrorArray Out"=w665:errorcluster[])  [unwired: 6 in, 1 out]
          }
          frame Enabled {
          }
        }
      }
      event User Event {
        w677 = TRUE ("Priority (F)")
        # "Queued Message Handler stops for any reason this top loop needs to also stop or an external stop call."
        n323 = event-data() -> ()  [unwired: 1 in, 1 out]
        n324 = call "Enqueue.vi"("Priority (F)"=w677, "ErrorArray"=w679, "Message"="Stop") -> ("ErrorArray"=w678:errorcluster[])  [unwired: 8 in]
      }
      event User Event {
        n325 = event-data() -> ("Data"=w684:variant)  [unwired: 1 in]
        n326 = call "InSSM.vi"() -> ("SSM State"=w681:bool)  [unwired: 11 in]
        n327 = case shown="False" w681 {
          tunnel: w684 -> [w690 _]
          tunnel: w683 -> [w688 w694]
          tunnel: [w687 w694] -> w682
          frame False {
            n328 = Variant To Data(type=errorcluster {"status"=FALSE, "code"=0, "source"=""} ("error constant"), Variant=w690) -> (data=w692:errorcluster, error out=w691:errorcluster)  [unwired: 1 in]
            n329 = Merge Errors(w692, w691) -> (w689:errorcluster)
            n330 = local read "Severity"() -> (w686:string)
            n331 = local read "Priority"() -> (w685:u8)
            n332 = call <userlib>:"AddError.vi"("Severity"=w686, "Priority"=w685, "ErrorArray In"=w688, "error in (no error)"=w689) -> ("ErrorArray Out"=w687:errorcluster[])  [unwired: 6 in, 1 out]
          }
          frame True {
          }
        }
      }
      event Pane Size {
        n333 = event-data() -> ()  [unwired: 1 in, 6 out]
        n334 = call "Enqueue.vi"("Message"="Center Logo") -> ("ErrorArray"=w695:errorcluster[])  [unwired: 10 in]
      }
      event "rngRunningModules": Value Change {
        n335 = event-data() -> ("NewVal"=w703:string)  [unwired: 1 in]
        n336 = call "VisualizationManager.vi"("Action"=VisualizationManagerActions."LoadModVI", "Module Name"=w703) -> ("error out"=w697:errorcluster, "In SubPanel?"=w698:bool)  [unwired: 6 in, 2 out]
        n337 = local write "btnPopOutModVis"(w698) -> ()
        n338 = call <userlib>:"AddError.vi"("Severity"="Critical", "Priority"=u8 2, "ErrorArray In"=w700, "error in (no error)"=w697) -> ("ErrorArray Out"=w699:errorcluster[])  [unwired: 6 in, 1 out]
      }
      event Value Change {
        n339 = event-data() -> ("NewVal"=w707:T1)  [unwired: 1 in]
        n340 = local read "rngRunningModules"() -> (w708:string)
        n341 = Bundle(cluster=cluster{"Module Name":string, "In SubPanel?":T1} {"Module Name"="", "In SubPanel?"=FALSE} ("output cluster"), "Module Name"=w708, "In SubPanel?"=w707) -> (w706:cluster{"Module Name":string, "In SubPanel?":T1})
        n342 = call "Enqueue.vi"("ErrorArray"=w711, "Message Data"=w706, "Message"="Pop In or Out of SubPanel") -> ("ErrorArray"=w710:errorcluster[])  [unwired: 8 in]
      }
      event "CurrentLogFile": Mouse Up {
        w715 = 128  # call and forget
        n343 = event-data() -> ()  [unwired: 1 in, 8 out]
        n344 = vi-ref <vilib>:"TDMS - File Viewer.vi"() -> (w714:refnum<vi>)
        n345 = property class="VI"(reference=w714) -> (error out=w722:errorcluster, "Name"=w721:string)  [unwired: 1 in, 1 out]
        n346 = Open VI Reference(type specifier VI Refnum (for type only)=refnum<vi> refnum, vi path=w721, options=w715, error in (no error)=w722) -> (vi reference=w717:refnum<vi>, error out=w712:errorcluster)  [unwired: 2 in]
        n347 = call "GetTDMSLogFilePath.vi"() -> ("TDMS Log File Path"=w713:path)  [unwired: 11 in]
        n348 = call-by-ref "Start Asynchronous Call"(reference=w717, error in=w712, 4:"error in (no error)"=w712, "file path"=w713) -> (reference out=w719:refnum<vi>, error out=w718:errorcluster)  [unwired: 4 in, 2 out]
        n349 = Close Reference(reference=w719, error in (no error)=w718) -> (error out=w720:errorcluster)
        n350 = call <vilib>:"Simple Error Handler.vi"("error in (no error)"=w720) -> ()  [unwired: 4 in, 5 out]
      }
      event "btnLoadTDMSData": Value Change {
        w728 = FALSE ("Wait Until Done")
        n351 = event-data() -> ()  [unwired: 1 in, 6 out]
        n352 = call <vilib>:"Application Directory.vi"() -> ("Application Directory"=w733:path)
        n353 = Build Path(base path=w733, name or relative path="NistPluggableModules\\Visualization\\StatusAndLog\\Status.vi") -> (appended path=w731:path)
        n354 = Open VI Reference(vi path=w731) -> (vi reference=w730:refnum<vi>, error out=w727:errorcluster)  [unwired: 5 in]
        n355 = invoke class="VI" method="FP.Open"(reference=w730, error in=w727, "Activate"=TRUE ("Activate?"), "State"=T23."Standard") -> (reference out=w729:refnum<vi>, error out=w726:errorcluster)  [unwired: 1 in, 3 out]
        n356 = invoke class="VI" method="Run VI"(reference=w729, error in=w726, "Wait until done"=w728, "Auto Dispose Ref"=w728) -> (error out=w723:errorcluster)  [unwired: 1 in, 4 out]
        n357 = call <vilib>:"Simple Error Handler.vi"("error in (no error)"=w723) -> ()  [unwired: 4 in, 5 out]
      }
      event "btnStopOneModule": Value Change {
        n358 = event-data() -> ()  [unwired: 1 in, 1 out]
        n359 = call "Enqueue.vi"("ErrorArray"=w734, "Message"="Stop One Module") -> ("ErrorArray"=w736:errorcluster[])  [unwired: 9 in]
      }
      event User Event {
        n360 = event-data() -> ("Module Name"=w745:string, "Data"=w744:variant)  [unwired: 1 in]
        n361 = Variant To Data(type=TRUE, Variant=w744) -> (data=w740:bool, error out=w738:errorcluster)  [unwired: 1 in]
        n362 = call <userlib>:"AddError.vi"("error in (no error)"=w738) -> ("ErrorArray Out"=w737:errorcluster[])  [unwired: 9 in, 1 out]
        n363 = Bundle(cluster=cluster{"Module Name":string, "In SubPanel?":T1} {"Module Name"="", "In SubPanel?"=FALSE} ("output cluster"), "Module Name"=w745, "In SubPanel?"=w740) -> (w742:cluster{"Module Name":string, "In SubPanel?":T1})
        n364 = call "Enqueue.vi"("ErrorArray"=w737, "Message Data"=w742, "Message"="Pop In or Out of SubPanel") -> ("ErrorArray"=w739:errorcluster[])  [unwired: 8 in]
      }
    }
    n365 = call "EnqueError.vi"("ErrorArrayIn"=w432) -> ("ErrorArrayOut"=w431:errorcluster[])  [unwired: 10 in]
  }
  n366 = call "Disconnect.vi"("ErrorArray"=w45) -> ("ErrorArray"=w36:errorcluster[])  [unwired: 10 in]
  n367 = Unregister For Events(event registration refnum=w7) -> (error out=w6:errorcluster)  [unwired: 1 in]
  n368 = call <userlib>:"AddError.vi"("Severity"="Fatal", "Priority"=u8 0, "ErrorArray In"=w31, "error in (no error)"=w6) -> ("ErrorArray Out"=w30:errorcluster[])  [unwired: 6 in, 1 out]
  n369 = Merge Errors(w30, w35, w36) -> (→"Error Out":errorcluster)
